vi "rs3_decode_streams.vi"(0 "Stream profile array":T2(array[cluster])=[{"ID"=42, "Profile"=521622968, "fps"=25, "RS Stream"=3, "RS Format"=10, "index"=2, "width"=1920, "height"=1080, "ppx"=0.0, "ppy"=0.0, "fx"=0.0, "fy"=0.0, "model"=0}, {"ID"=41, "Profile"=521634232, "fps"=25, "RS Stream"=3, "RS Format"=10, "index"=1, "width"=1920, "height"=1080, "ppx"=0.0, "ppy"=0.0, "fx"=0.0, "fy"=0.0, "model"=0}, {"ID"=42, "Profile"=521608632, "fps"=25, "RS Stream"=3, "RS Format"=9, "index"=2, "width"=1920, "height"=1080, "ppx"=951.85925, "ppy"=556.0496, "fx"=1428.9095, "fy"=1428.9095, "model"=4}, {"ID"=41, "Profile"=521617080, "fps"=25, "RS Stream"=3, "RS Format"=9, "index"=1, "width"=1920, "height"=1080, "ppx"=951.85925, "ppy"=556.0496, "fx"=1428.9095, "fy"=1428.9095, "model"=4}, {"ID"=41, "Profile"=521619128, "fps"=15, "RS Stream"=3, "RS Format"=10, "index"=1, "width"=1920, "height"=1080, "ppx"=0.0, "ppy"=0.0, "fx"=0.0, "fy"=0.0, "model"=0}, {"ID"=42, "Profile"=521623224, "fps"=15, "RS Stream"=3, "RS Format"=10, "index"=2, "width"=1920, "height"=1080, "ppx"=0.0, "ppy"=0.0, "fx"=0.0, "fy"=0.0, "model"=0}, {"ID"=42, "Profile"=521628088, "fps"=15, "RS Stream"=3, "RS Format"=9, "index"=2, "width"=1920, "height"=1080, "ppx"=951.85925, "ppy"=556.0496, "fx"=1428.9095, "fy"=1428.9095, "model"=4}, {"ID"=41, "Profile"=521627576, "fps"=15, "RS Stream"=3, "RS Format"=9, "index"=1, "width"=1920, "height"=1080, "ppx"=951.85925, "ppy"=556.0496, "fx"=1428.9095, "fy"=1428.9095, "model"=4}, {"ID"=41, "Profile"=521612728, "fps"=30, "RS Stream"=3, "RS Format"=14, "index"=0, "width"=1280, "height"=720, "ppx"=634.5728, "ppy"=370.69974, "fx"=952.6064, "fy"=952.6064, "model"=4}, {"ID"=41, "Profile"=521610424, "fps"=30, "RS Stream"=3, "RS Format"=10, "index"=0, "width"=1280, "height"=720, "ppx"=0.0, "ppy"=0.0, "fx"=0.0, "fy"=0.0, "model"=0}, {"ID"=42, "Profile"=521615544, "fps"=30, "RS Stream"=3, "RS Format"=9, "index"=2, "width"=1280, "height"=720, "ppx"=634.5728, "ppy"=370.69974, "fx"=952.6064, "fy"=952.6064, "model"=4}, {"ID"=41, "Profile"=521320344, "fps"=30, "RS Stream"=3, "RS Format"=9, "index"=1, "width"=1280, "height"=720, "ppx"=634.5728, "ppy"=370.69974, "fx"=952.6064, "fy"=952.6064, "model"=4}, {"ID"=41, "Profile"=521614520, "fps"=30, "RS Stream"=3, "RS Format"=8, "index"=0, "width"=1280, "height"=720, "ppx"=634.5728, "ppy"=370.69974, "fx"=952.6064, "fy"=952.6064, "model"=4}, {"ID"=41, "Profile"=521605816, "fps"=30, "RS Stream"=3, "RS Format"=7, "index"=0, "width"=1280, "height"=720, "ppx"=634.5728, "ppy"=370.69974, "fx"=952.6064, "fy"=952.6064, "model"=4}, {"ID"=41, "Profile"=521607608, "fps"=30, "RS Stream"=3, "RS Format"=6, "index"=0, "width"=1280, "height"=720, "ppx"=634.5728, "ppy"=370.69974, "fx"=952.6064, "fy"=952.6064, "model"=4}, {"ID"=41, "Profile"=521605560, "fps"=30, "RS Stream"=3, "RS Format"=5, "index"=0, "width"=1280, "height"=720, "ppx"=634.5728, "ppy"=370.69974, "fx"=952.6064, "fy"=952.6064, "model"=4}, {"ID"=41, "Profile"=521609912, "fps"=15, "RS Stream"=3, "RS Format"=14, "index"=0, "width"=1280, "height"=720, "ppx"=634.5728, "ppy"=370.69974, "fx"=952.6064, "fy"=952.6064, "model"=4}, {"ID"=41, "Profile"=521606584, "fps"=15, "RS Stream"=3, "RS Format"=10, "index"=0, "width"=1280, "height"=720, "ppx"=0.0, "ppy"=0.0, "fx"=0.0, "fy"=0.0, "model"=0}, {"ID"=41, "Profile"=521310872, "fps"=15, "RS Stream"=3, "RS Format"=9, "index"=1, "width"=1280, "height"=720, "ppx"=634.5728, "ppy"=370.69974, "fx"=952.6064, "fy"=952.6064, "model"=4}, {"ID"=42, "Profile"=521616824, "fps"=15, "RS Stream"=3, "RS Format"=9, "index"=2, "width"=1280, "height"=720, "ppx"=634.5728, "ppy"=370.69974, "fx"=952.6064, "fy"=952.6064, "model"=4}, {"ID"=41, "Profile"=521604024, "fps"=15, "RS Stream"=3, "RS Format"=8, "index"=0, "width"=1280, "height"=720, "ppx"=634.5728, "ppy"=370.69974, "fx"=952.6064, "fy"=952.6064, "model"=4}, {"ID"=41, "Profile"=521612984, "fps"=15, "RS Stream"=3, "RS Format"=7, "index"=0, "width"=1280, "height"=720, "ppx"=634.5728, "ppy"=370.69974, "fx"=952.6064, "fy"=952.6064, "model"=4}, {"ID"=41, "Profile"=521610168, "fps"=15, "RS Stream"=3, "RS Format"=6, "index"=0, "width"=1280, "height"=720, "ppx"=634.5728, "ppy"=370.69974, "fx"=952.6064, "fy"=952.6064, "model"=4}, {"ID"=41, "Profile"=521604536, "fps"=15, "RS Stream"=3, "RS Format"=5, "index"=0, "width"=1280, "height"=720, "ppx"=634.5728, "ppy"=370.69974, "fx"=952.6064, "fy"=952.6064, "model"=4}, {"ID"=41, "Profile"=521617848, "fps"=6, "RS Stream"=3, "RS Format"=14, "index"=0, "width"=1280, "height"=720, "ppx"=634.5728, "ppy"=370.69974, "fx"=952.6064, "fy"=952.6064, "model"=4}, {"ID"=41, "Profile"=521613752, "fps"=6, "RS Stream"=3, "RS Format"=10, "index"=0, "width"=1280, "height"=720, "ppx"=0.0, "ppy"=0.0, "fx"=0.0, "fy"=0.0, "model"=0}, {"ID"=41, "Profile"=521320600, "fps"=6, "RS Stream"=3, "RS Format"=9, "index"=1, "width"=1280, "height"=720, "ppx"=634.5728, "ppy"=370.69974, "fx"=952.6064, "fy"=952.6064, "model"=4}, {"ID"=42, "Profile"=521608888, "fps"=6, "RS Stream"=3, "RS Format"=9, "index"=2, "width"=1280, "height"=720, "ppx"=634.5728, "ppy"=370.69974, "fx"=952.6064, "fy"=952.6064, "model"=4}, {"ID"=41, "Profile"=521613240, "fps"=6, "RS Stream"=3, "RS Format"=8, "index"=0, "width"=1280, "height"=720, "ppx"=634.5728, "ppy"=370.69974, "fx"=952.6064, "fy"=952.6064, "model"=4}, {"ID"=41, "Profile"=521611704, "fps"=6, "RS Stream"=3, "RS Format"=7, "index"=0, "width"=1280, "height"=720, "ppx"=634.5728, "ppy"=370.69974, "fx"=952.6064, "fy"=952.6064, "model"=4}, {"ID"=41, "Profile"=521601720, "fps"=6, "RS Stream"=3, "RS Format"=6, "index"=0, "width"=1280, "height"=720, "ppx"=634.5728, "ppy"=370.69974, "fx"=952.6064, "fy"=952.6064, "model"=4}, {"ID"=41, "Profile"=521617336, "fps"=6, "RS Stream"=3, "RS Format"=5, "index"=0, "width"=1280, "height"=720, "ppx"=634.5728, "ppy"=370.69974, "fx"=952.6064, "fy"=952.6064, "model"=4}, {"ID"=41, "Profile"=521622712, "fps"=25, "RS Stream"=3, "RS Format"=10, "index"=1, "width"=960, "height"=540, "ppx"=0.0, "ppy"=0.0, "fx"=0.0, "fy"=0.0, "model"=0}, {"ID"=42, "Profile"=521633976, "fps"=25, "RS Stream"=3, "RS Format"=10, "index"=2, "width"=960, "height"=540, "ppx"=0.0, "ppy"=0.0, "fx"=0.0, "fy"=0.0, "model"=0}, {"ID"=42, "Profile"=521624504, "fps"=15, "RS Stream"=3, "RS Format"=10, "index"=2, "width"=960, "height"=540, "ppx"=0.0, "ppy"=0.0, "fx"=0.0, "fy"=0.0, "model"=0}, {"ID"=41, "Profile"=521622456, "fps"=15, "RS Stream"=3, "RS Format"=10, "index"=1, "width"=960, "height"=540, "ppx"=0.0, "ppy"=0.0, "fx"=0.0, "fy"=0.0, "model"=0}, {"ID"=41, "Profile"=521352856, "fps"=90, "RS Stream"=3, "RS Format"=14, "index"=0, "width"=848, "height"=480, "ppx"=420.38187, "ppy"=247.13316, "fx"=635.0709, "fy"=635.0709, "model"=4}, {"ID"=41, "Profile"=521351320, "fps"=90, "RS Stream"=3, "RS Format"=10, "index"=0, "width"=848, "height"=480, "ppx"=0.0, "ppy"=0.0, "fx"=0.0, "fy"=0.0, "model"=0}, {"ID"=41, "Profile"=521306776, "fps"=90, "RS Stream"=3, "RS Format"=9, "index"=1, "width"=848, "height"=480, "ppx"=420.38187, "ppy"=247.13316, "fx"=635.0709, "fy"=635.0709, "model"=4}, {"ID"=42, "Profile"=521614776, "fps"=90, "RS Stream"=3, "RS Format"=9, "index"=2, "width"=848, "height"=480, "ppx"=420.38187, "ppy"=247.13316, "fx"=635.0709, "fy"=635.0709, "model"=4}, {"ID"=41, "Profile"=521353624, "fps"=90, "RS Stream"=3, "RS Format"=8, "index"=0, "width"=848, "height"=480, "ppx"=420.38187, "ppy"=247.13316, "fx"=635.0709, "fy"=635.0709, "model"=4}, {"ID"=41, "Profile"=521339544, "fps"=90, "RS Stream"=3, "RS Format"=7, "index"=0, "width"=848, "height"=480, "ppx"=420.38187, "ppy"=247.13316, "fx"=635.0709, "fy"=635.0709, "model"=4}, {"ID"=41, "Profile"=521353368, "fps"=90, "RS Stream"=3, "RS Format"=6, "index"=0, "width"=848, "height"=480, "ppx"=420.38187, "ppy"=247.13316, "fx"=635.0709, "fy"=635.0709, "model"=4}, {"ID"=41, "Profile"=521351064, "fps"=90, "RS Stream"=3, "RS Format"=5, "index"=0, "width"=848, "height"=480, "ppx"=420.38187, "ppy"=247.13316, "fx"=635.0709, "fy"=635.0709, "model"=4}, {"ID"=41, "Profile"=521342104, "fps"=60, "RS Stream"=3, "RS Format"=14, "index"=0, "width"=848, "height"=480, "ppx"=420.38187, "ppy"=247.13316, "fx"=635.0709, "fy"=635.0709, "model"=4}, {"ID"=41, "Profile"=521341848, "fps"=60, "RS Stream"=3, "RS Format"=10, "index"=0, "width"=848, "height"=480, "ppx"=0.0, "ppy"=0.0, "fx"=0.0, "fy"=0.0, "model"=0}, {"ID"=42, "Profile"=521611960, "fps"=60, "RS Stream"=3, "RS Format"=9, "index"=2, "width"=848, "height"=480, "ppx"=420.38187, "ppy"=247.13316, "fx"=635.0709, "fy"=635.0709, "model"=4}, {"ID"=41, "Profile"=521310360, "fps"=60, "RS Stream"=3, "RS Format"=9, "index"=1, "width"=848, "height"=480, "ppx"=420.38187, "ppy"=247.13316, "fx"=635.0709, "fy"=635.0709, "model"=4}, {"ID"=41, "Profile"=521343384, "fps"=60, "RS Stream"=3, "RS Format"=8, "index"=0, "width"=848, "height"=480, "ppx"=420.38187, "ppy"=247.13316, "fx"=635.0709, "fy"=635.0709, "model"=4}, {"ID"=41, "Profile"=521342360, "fps"=60, "RS Stream"=3, "RS Format"=7, "index"=0, "width"=848, "height"=480, "ppx"=420.38187, "ppy"=247.13316, "fx"=635.0709, "fy"=635.0709, "model"=4}, {"ID"=41, "Profile"=521342616, "fps"=60, "RS Stream"=3, "RS Format"=6, "index"=0, "width"=848, "height"=480, "ppx"=420.38187, "ppy"=247.13316, "fx"=635.0709, "fy"=635.0709, "model"=4}, {"ID"=41, "Profile"=521354136, "fps"=60, "RS Stream"=3, "RS Format"=5, "index"=0, "width"=848, "height"=480, "ppx"=420.38187, "ppy"=247.13316, "fx"=635.0709, "fy"=635.0709, "model"=4}, {"ID"=41, "Profile"=521616056, "fps"=30, "RS Stream"=3, "RS Format"=14, "index"=0, "width"=848, "height"=480, "ppx"=420.38187, "ppy"=247.13316, "fx"=635.0709, "fy"=635.0709, "model"=4}, {"ID"=41, "Profile"=514733800, "fps"=30, "RS Stream"=3, "RS Format"=10, "index"=0, "width"=848, "height"=480, "ppx"=0.0, "ppy"=0.0, "fx"=0.0, "fy"=0.0, "model"=0}, {"ID"=42, "Profile"=521609144, "fps"=30, "RS Stream"=3, "RS Format"=9, "index"=2, "width"=848, "height"=480, "ppx"=420.38187, "ppy"=247.13316, "fx"=635.0709, "fy"=635.0709, "model"=4}, {"ID"=41, "Profile"=521310616, "fps"=30, "RS Stream"=3, "RS Format"=9, "index"=1, "width"=848, "height"=480, "ppx"=420.38187, "ppy"=247.13316, "fx"=635.0709, "fy"=635.0709, "model"=4}, {"ID"=41, "Profile"=521606840, "fps"=30, "RS Stream"=3, "RS Format"=8, "index"=0, "width"=848, "height"=480, "ppx"=420.38187, "ppy"=247.13316, "fx"=635.0709, "fy"=635.0709, "model"=4}, {"ID"=41, "Profile"=521603256, "fps"=30, "RS Stream"=3, "RS Format"=7, "index"=0, "width"=848, "height"=480, "ppx"=420.38187, "ppy"=247.13316, "fx"=635.0709, "fy"=635.0709, "model"=4}, {"ID"=41, "Profile"=521612472, "fps"=30, "RS Stream"=3, "RS Format"=6, "index"=0, "width"=848, "height"=480, "ppx"=420.38187, "ppy"=247.13316, "fx"=635.0709, "fy"=635.0709, "model"=4}, {"ID"=41, "Profile"=521343640, "fps"=30, "RS Stream"=3, "RS Format"=5, "index"=0, "width"=848, "height"=480, "ppx"=420.38187, "ppy"=247.13316, "fx"=635.0709, "fy"=635.0709, "model"=4}, {"ID"=41, "Profile"=521609400, "fps"=15, "RS Stream"=3, "RS Format"=14, "index"=0, "width"=848, "height"=480, "ppx"=420.38187, "ppy"=247.13316, "fx"=635.0709, "fy"=635.0709, "model"=4}, {"ID"=41, "Profile"=521606328, "fps"=15, "RS Stream"=3, "RS Format"=10, "index"=0, "width"=848, "height"=480, "ppx"=0.0, "ppy"=0.0, "fx"=0.0, "fy"=0.0, "model"=0}, {"ID"=41, "Profile"=521317272, "fps"=15, "RS Stream"=3, "RS Format"=9, "index"=1, "width"=848, "height"=480, "ppx"=420.38187, "ppy"=247.13316, "fx"=635.0709, "fy"=635.0709, "model"=4}, {"ID"=42, "Profile"=521615288, "fps"=15, "RS Stream"=3, "RS Format"=9, "index"=2, "width"=848, "height"=480, "ppx"=420.38187, "ppy"=247.13316, "fx"=635.0709, "fy"=635.0709, "model"=4}, {"ID"=41, "Profile"=521603512, "fps"=15, "RS Stream"=3, "RS Format"=8, "index"=0, "width"=848, "height"=480, "ppx"=420.38187, "ppy"=247.13316, "fx"=635.0709, "fy"=635.0709, "model"=4}, {"ID"=41, "Profile"=521602744, "fps"=15, "RS Stream"=3, "RS Format"=7, "index"=0, "width"=848, "height"=480, "ppx"=420.38187, "ppy"=247.13316, "fx"=635.0709, "fy"=635.0709, "model"=4}, {"ID"=41, "Profile"=521607096, "fps"=15, "RS Stream"=3, "RS Format"=6, "index"=0, "width"=848, "height"=480, "ppx"=420.38187, "ppy"=247.13316, "fx"=635.0709, "fy"=635.0709, "model"=4}, {"ID"=41, "Profile"=521617592, "fps"=15, "RS Stream"=3, "RS Format"=5, "index"=0, "width"=848, "height"=480, "ppx"=420.38187, "ppy"=247.13316, "fx"=635.0709, "fy"=635.0709, "model"=4}, {"ID"=41, "Profile"=521603768, "fps"=6, "RS Stream"=3, "RS Format"=14, "index"=0, "width"=848, "height"=480, "ppx"=420.38187, "ppy"=247.13316, "fx"=635.0709, "fy"=635.0709, "model"=4}, {"ID"=41, "Profile"=521604280, "fps"=6, "RS Stream"=3, "RS Format"=10, "index"=0, "width"=848, "height"=480, "ppx"=0.0, "ppy"=0.0, "fx"=0.0, "fy"=0.0, "model"=0}, {"ID"=42, "Profile"=521616568, "fps"=6, "RS Stream"=3, "RS Format"=9, "index"=2, "width"=848, "height"=480, "ppx"=420.38187, "ppy"=247.13316, "fx"=635.0709, "fy"=635.0709, "model"=4}, {"ID"=41, "Profile"=521315992, "fps"=6, "RS Stream"=3, "RS Format"=9, "index"=1, "width"=848, "height"=480, "ppx"=420.38187, "ppy"=247.13316, "fx"=635.0709, "fy"=635.0709, "model"=4}, {"ID"=41, "Profile"=521607864, "fps"=6, "RS Stream"=3, "RS Format"=8, "index"=0, "width"=848, "height"=480, "ppx"=420.38187, "ppy"=247.13316, "fx"=635.0709, "fy"=635.0709, "model"=4}, {"ID"=41, "Profile"=521616312, "fps"=6, "RS Stream"=3, "RS Format"=7, "index"=0, "width"=848, "height"=480, "ppx"=420.38187, "ppy"=247.13316, "fx"=635.0709, "fy"=635.0709, "model"=4}, {"ID"=41, "Profile"=521615800, "fps"=6, "RS Stream"=3, "RS Format"=6, "index"=0, "width"=848, "height"=480, "ppx"=420.38187, "ppy"=247.13316, "fx"=635.0709, "fy"=635.0709, "model"=4}, {"ID"=41, "Profile"=521610680, "fps"=6, "RS Stream"=3, "RS Format"=5, "index"=0, "width"=848, "height"=480, "ppx"=420.38187, "ppy"=247.13316, "fx"=635.0709, "fy"=635.0709, "model"=4}, {"ID"=41, "Profile"=521348504, "fps"=90, "RS Stream"=3, "RS Format"=14, "index"=0, "width"=640, "height"=480, "ppx"=316.38187, "ppy"=247.13316, "fx"=635.0709, "fy"=635.0709, "model"=4}, {"ID"=41, "Profile"=521354904, "fps"=90, "RS Stream"=3, "RS Format"=10, "index"=0, "width"=640, "height"=480, "ppx"=0.0, "ppy"=0.0, "fx"=0.0, "fy"=0.0, "model"=0}, {"ID"=42, "Profile"=521605304, "fps"=90, "RS Stream"=3, "RS Format"=9, "index"=2, "width"=640, "height"=480, "ppx"=316.38187, "ppy"=247.13316, "fx"=635.0709, "fy"=635.0709, "model"=4}, {"ID"=41, "Profile"=521322648, "fps"=90, "RS Stream"=3, "RS Format"=9, "index"=1, "width"=640, "height"=480, "ppx"=316.38187, "ppy"=247.13316, "fx"=635.0709, "fy"=635.0709, "model"=4}, {"ID"=41, "Profile"=521340056, "fps"=90, "RS Stream"=3, "RS Format"=8, "index"=0, "width"=640, "height"=480, "ppx"=316.38187, "ppy"=247.13316, "fx"=635.0709, "fy"=635.0709, "model"=4}, {"ID"=41, "Profile"=521355672, "fps"=90, "RS Stream"=3, "RS Format"=7, "index"=0, "width"=640, "height"=480, "ppx"=316.38187, "ppy"=247.13316, "fx"=635.0709, "fy"=635.0709, "model"=4}, {"ID"=41, "Profile"=521352088, "fps"=90, "RS Stream"=3, "RS Format"=6, "index"=0, "width"=640, "height"=480, "ppx"=316.38187, "ppy"=247.13316, "fx"=635.0709, "fy"=635.0709, "model"=4}, {"ID"=41, "Profile"=521351576, "fps"=90, "RS Stream"=3, "RS Format"=5, "index"=0, "width"=640, "height"=480, "ppx"=316.38187, "ppy"=247.13316, "fx"=635.0709, "fy"=635.0709, "model"=4}, {"ID"=41, "Profile"=521352344, "fps"=60, "RS Stream"=3, "RS Format"=14, "index"=0, "width"=640, "height"=480, "ppx"=316.38187, "ppy"=247.13316, "fx"=635.0709, "fy"=635.0709, "model"=4}, {"ID"=41, "Profile"=521354648, "fps"=60, "RS Stream"=3, "RS Format"=10, "index"=0, "width"=640, "height"=480, "ppx"=0.0, "ppy"=0.0, "fx"=0.0, "fy"=0.0, "model"=0}, {"ID"=41, "Profile"=521320088, "fps"=60, "RS Stream"=3, "RS Format"=9, "index"=1, "width"=640, "height"=480, "ppx"=316.38187, "ppy"=247.13316, "fx"=635.0709, "fy"=635.0709, "model"=4}, {"ID"=42, "Profile"=521615032, "fps"=60, "RS Stream"=3, "RS Format"=9, "index"=2, "width"=640, "height"=480, "ppx"=316.38187, "ppy"=247.13316, "fx"=635.0709, "fy"=635.0709, "model"=4}, {"ID"=41, "Profile"=521340312, "fps"=60, "RS Stream"=3, "RS Format"=8, "index"=0, "width"=640, "height"=480, "ppx"=316.38187, "ppy"=247.13316, "fx"=635.0709, "fy"=635.0709, "model"=4}, {"ID"=41, "Profile"=521342872, "fps"=60, "RS Stream"=3, "RS Format"=7, "index"=0, "width"=640, "height"=480, "ppx"=316.38187, "ppy"=247.13316, "fx"=635.0709, "fy"=635.0709, "model"=4}, {"ID"=41, "Profile"=521346200, "fps"=60, "RS Stream"=3, "RS Format"=6, "index"=0, "width"=640, "height"=480, "ppx"=316.38187, "ppy"=247.13316, "fx"=635.0709, "fy"=635.0709, "model"=4}, {"ID"=41, "Profile"=521345944, "fps"=60, "RS Stream"=3, "RS Format"=5, "index"=0, "width"=640, "height"=480, "ppx"=316.38187, "ppy"=247.13316, "fx"=635.0709, "fy"=635.0709, "model"=4}, {"ID"=41, "Profile"=521344408, "fps"=30, "RS Stream"=3, "RS Format"=14, "index"=0, "width"=640, "height"=480, "ppx"=316.38187, "ppy"=247.13316, "fx"=635.0709, "fy"=635.0709, "model"=4}, {"ID"=41, "Profile"=521348248, "fps"=30, "RS Stream"=3, "RS Format"=10, "index"=0, "width"=640, "height"=480, "ppx"=0.0, "ppy"=0.0, "fx"=0.0, "fy"=0.0, "model"=0}, {"ID"=41, "Profile"=521309592, "fps"=30, "RS Stream"=3, "RS Format"=9, "index"=1, "width"=640, "height"=480, "ppx"=316.38187, "ppy"=247.13316, "fx"=635.0709, "fy"=635.0709, "model"=4}, {"ID"=42, "Profile"=521607352, "fps"=30, "RS Stream"=3, "RS Format"=9, "index"=2, "width"=640, "height"=480, "ppx"=316.38187, "ppy"=247.13316, "fx"=635.0709, "fy"=635.0709, "model"=4}, {"ID"=41, "Profile"=521352600, "fps"=30, "RS Stream"=3, "RS Format"=8, "index"=0, "width"=640, "height"=480, "ppx"=316.38187, "ppy"=247.13316, "fx"=635.0709, "fy"=635.0709, "model"=4}, {"ID"=41, "Profile"=521344664, "fps"=30, "RS Stream"=3, "RS Format"=7, "index"=0, "width"=640, "height"=480, "ppx"=316.38187, "ppy"=247.13316, "fx"=635.0709, "fy"=635.0709, "model"=4}, {"ID"=41, "Profile"=521344920, "fps"=30, "RS Stream"=3, "RS Format"=6, "index"=0, "width"=640, "height"=480, "ppx"=316.38187, "ppy"=247.13316, "fx"=635.0709, "fy"=635.0709, "model"=4}, {"ID"=41, "Profile"=521350296, "fps"=30, "RS Stream"=3, "RS Format"=5, "index"=0, "width"=640, "height"=480, "ppx"=316.38187, "ppy"=247.13316, "fx"=635.0709, "fy"=635.0709, "model"=4}, {"ID"=41, "Profile"=521355160, "fps"=15, "RS Stream"=3, "RS Format"=14, "index"=0, "width"=640, "height"=480, "ppx"=316.38187, "ppy"=247.13316, "fx"=635.0709, "fy"=635.0709, "model"=4}, {"ID"=41, "Profile"=521341592, "fps"=15, "RS Stream"=3, "RS Format"=10, "index"=0, "width"=640, "height"=480, "ppx"=0.0, "ppy"=0.0, "fx"=0.0, "fy"=0.0, "model"=0}, {"ID"=41, "Profile"=521321368, "fps"=15, "RS Stream"=3, "RS Format"=9, "index"=1, "width"=640, "height"=480, "ppx"=316.38187, "ppy"=247.13316, "fx"=635.0709, "fy"=635.0709, "model"=4}, {"ID"=42, "Profile"=521608120, "fps"=15, "RS Stream"=3, "RS Format"=9, "index"=2, "width"=640, "height"=480, "ppx"=316.38187, "ppy"=247.13316, "fx"=635.0709, "fy"=635.0709, "model"=4}, {"ID"=41, "Profile"=521346968, "fps"=15, "RS Stream"=3, "RS Format"=8, "index"=0, "width"=640, "height"=480, "ppx"=316.38187, "ppy"=247.13316, "fx"=635.0709, "fy"=635.0709, "model"=4}, {"ID"=41, "Profile"=521348760, "fps"=15, "RS Stream"=3, "RS Format"=7, "index"=0, "width"=640, "height"=480, "ppx"=316.38187, "ppy"=247.13316, "fx"=635.0709, "fy"=635.0709, "model"=4}, {"ID"=41, "Profile"=521339800, "fps"=15, "RS Stream"=3, "RS Format"=6, "index"=0, "width"=640, "height"=480, "ppx"=316.38187, "ppy"=247.13316, "fx"=635.0709, "fy"=635.0709, "model"=4}, {"ID"=41, "Profile"=521350808, "fps"=15, "RS Stream"=3, "RS Format"=5, "index"=0, "width"=640, "height"=480, "ppx"=316.38187, "ppy"=247.13316, "fx"=635.0709, "fy"=635.0709, "model"=4}, {"ID"=41, "Profile"=521349016, "fps"=6, "RS Stream"=3, "RS Format"=14, "index"=0, "width"=640, "height"=480, "ppx"=316.38187, "ppy"=247.13316, "fx"=635.0709, "fy"=635.0709, "model"=4}, {"ID"=41, "Profile"=521346456, "fps"=6, "RS Stream"=3, "RS Format"=10, "index"=0, "width"=640, "height"=480, "ppx"=0.0, "ppy"=0.0, "fx"=0.0, "fy"=0.0, "model"=0}, {"ID"=42, "Profile"=521608376, "fps"=6, "RS Stream"=3, "RS Format"=9, "index"=2, "width"=640, "height"=480, "ppx"=316.38187, "ppy"=247.13316, "fx"=635.0709, "fy"=635.0709, "model"=4}, {"ID"=41, "Profile"=521313176, "fps"=6, "RS Stream"=3, "RS Format"=9, "index"=1, "width"=640, "height"=480, "ppx"=316.38187, "ppy"=247.13316, "fx"=635.0709, "fy"=635.0709, "model"=4}, {"ID"=41, "Profile"=521343128, "fps"=6, "RS Stream"=3, "RS Format"=8, "index"=0, "width"=640, "height"=480, "ppx"=316.38187, "ppy"=247.13316, "fx"=635.0709, "fy"=635.0709, "model"=4}, {"ID"=41, "Profile"=521349528, "fps"=6, "RS Stream"=3, "RS Format"=7, "index"=0, "width"=640, "height"=480, "ppx"=316.38187, "ppy"=247.13316, "fx"=635.0709, "fy"=635.0709, "model"=4}, {"ID"=41, "Profile"=521355416, "fps"=6, "RS Stream"=3, "RS Format"=6, "index"=0, "width"=640, "height"=480, "ppx"=316.38187, "ppy"=247.13316, "fx"=635.0709, "fy"=635.0709, "model"=4}, {"ID"=41, "Profile"=521349272, "fps"=6, "RS Stream"=3, "RS Format"=5, "index"=0, "width"=640, "height"=480, "ppx"=316.38187, "ppy"=247.13316, "fx"=635.0709, "fy"=635.0709, "model"=4}, {"ID"=41, "Profile"=521330840, "fps"=90, "RS Stream"=3, "RS Format"=14, "index"=0, "width"=640, "height"=360, "ppx"=317.2864, "ppy"=185.34987, "fx"=476.3032, "fy"=476.3032, "model"=4}, {"ID"=41, "Profile"=521330584, "fps"=90, "RS Stream"=3, "RS Format"=10, "index"=0, "width"=640, "height"=360, "ppx"=0.0, "ppy"=0.0, "fx"=0.0, "fy"=0.0, "model"=0}, {"ID"=41, "Profile"=521318296, "fps"=90, "RS Stream"=3, "RS Format"=9, "index"=1, "width"=640, "height"=360, "ppx"=317.2864, "ppy"=185.34987, "fx"=476.3032, "fy"=476.3032, "model"=4}, {"ID"=42, "Profile"=521609656, "fps"=90, "RS Stream"=3, "RS Format"=9, "index"=2, "width"=640, "height"=360, "ppx"=317.2864, "ppy"=185.34987, "fx"=476.3032, "fy"=476.3032, "model"=4}, {"ID"=41, "Profile"=521332120, "fps"=90, "RS Stream"=3, "RS Format"=8, "index"=0, "width"=640, "height"=360, "ppx"=317.2864, "ppy"=185.34987, "fx"=476.3032, "fy"=476.3032, "model"=4}, {"ID"=41, "Profile"=521331608, "fps"=90, "RS Stream"=3, "RS Format"=7, "index"=0, "width"=640, "height"=360, "ppx"=317.2864, "ppy"=185.34987, "fx"=476.3032, "fy"=476.3032, "model"=4}, {"ID"=41, "Profile"=521331864, "fps"=90, "RS Stream"=3, "RS Format"=6, "index"=0, "width"=640, "height"=360, "ppx"=317.2864, "ppy"=185.34987, "fx"=476.3032, "fy"=476.3032, "model"=4}, {"ID"=41, "Profile"=521326744, "fps"=90, "RS Stream"=3, "RS Format"=5, "index"=0, "width"=640, "height"=360, "ppx"=317.2864, "ppy"=185.34987, "fx"=476.3032, "fy"=476.3032, "model"=4}, {"ID"=41, "Profile"=521333912, "fps"=60, "RS Stream"=3, "RS Format"=14, "index"=0, "width"=640, "height"=360, "ppx"=317.2864, "ppy"=185.34987, "fx"=476.3032, "fy"=476.3032, "model"=4}, {"ID"=41, "Profile"=521333144, "fps"=60, "RS Stream"=3, "RS Format"=10, "index"=0, "width"=640, "height"=360, "ppx"=0.0, "ppy"=0.0, "fx"=0.0, "fy"=0.0, "model"=0}, {"ID"=42, "Profile"=521606072, "fps"=60, "RS Stream"=3, "RS Format"=9, "index"=2, "width"=640, "height"=360, "ppx"=317.2864, "ppy"=185.34987, "fx"=476.3032, "fy"=476.3032, "model"=4}, {"ID"=41, "Profile"=521321112, "fps"=60, "RS Stream"=3, "RS Format"=9, "index"=1, "width"=640, "height"=360, "ppx"=317.2864, "ppy"=185.34987, "fx"=476.3032, "fy"=476.3032, "model"=4}, {"ID"=41, "Profile"=521340824, "fps"=60, "RS Stream"=3, "RS Format"=8, "index"=0, "width"=640, "height"=360, "ppx"=317.2864, "ppy"=185.34987, "fx"=476.3032, "fy"=476.3032, "model"=4}, {"ID"=41, "Profile"=521353880, "fps"=60, "RS Stream"=3, "RS Format"=7, "index"=0, "width"=640, "height"=360, "ppx"=317.2864, "ppy"=185.34987, "fx"=476.3032, "fy"=476.3032, "model"=4}, {"ID"=41, "Profile"=521350552, "fps"=60, "RS Stream"=3, "RS Format"=6, "index"=0, "width"=640, "height"=360, "ppx"=317.2864, "ppy"=185.34987, "fx"=476.3032, "fy"=476.3032, "model"=4}, {"ID"=41, "Profile"=521332888, "fps"=60, "RS Stream"=3, "RS Format"=5, "index"=0, "width"=640, "height"=360, "ppx"=317.2864, "ppy"=185.34987, "fx"=476.3032, "fy"=476.3032, "model"=4}, {"ID"=41, "Profile"=521347224, "fps"=30, "RS Stream"=3, "RS Format"=14, "index"=0, "width"=640, "height"=360, "ppx"=317.2864, "ppy"=185.34987, "fx"=476.3032, "fy"=476.3032, "model"=4}, {"ID"=41, "Profile"=521349784, "fps"=30, "RS Stream"=3, "RS Format"=10, "index"=0, "width"=640, "height"=360, "ppx"=0.0, "ppy"=0.0, "fx"=0.0, "fy"=0.0, "model"=0}, {"ID"=42, "Profile"=521604792, "fps"=30, "RS Stream"=3, "RS Format"=9, "index"=2, "width"=640, "height"=360, "ppx"=317.2864, "ppy"=185.34987, "fx"=476.3032, "fy"=476.3032, "model"=4}, {"ID"=41, "Profile"=521319064, "fps"=30, "RS Stream"=3, "RS Format"=9, "index"=1, "width"=640, "height"=360, "ppx"=317.2864, "ppy"=185.34987, "fx"=476.3032, "fy"=476.3032, "model"=4}, {"ID"=41, "Profile"=521351832, "fps"=30, "RS Stream"=3, "RS Format"=8, "index"=0, "width"=640, "height"=360, "ppx"=317.2864, "ppy"=185.34987, "fx"=476.3032, "fy"=476.3032, "model"=4}, {"ID"=41, "Profile"=521347480, "fps"=30, "RS Stream"=3, "RS Format"=7, "index"=0, "width"=640, "height"=360, "ppx"=317.2864, "ppy"=185.34987, "fx"=476.3032, "fy"=476.3032, "model"=4}, {"ID"=41, "Profile"=521350040, "fps"=30, "RS Stream"=3, "RS Format"=6, "index"=0, "width"=640, "height"=360, "ppx"=317.2864, "ppy"=185.34987, "fx"=476.3032, "fy"=476.3032, "model"=4}, {"ID"=41, "Profile"=521345432, "fps"=30, "RS Stream"=3, "RS Format"=5, "index"=0, "width"=640, "height"=360, "ppx"=317.2864, "ppy"=185.34987, "fx"=476.3032, "fy"=476.3032, "model"=4}, {"ID"=41, "Profile"=521343896, "fps"=15, "RS Stream"=3, "RS Format"=14, "index"=0, "width"=640, "height"=360, "ppx"=317.2864, "ppy"=185.34987, "fx"=476.3032, "fy"=476.3032, "model"=4}, {"ID"=41, "Profile"=521340568, "fps"=15, "RS Stream"=3, "RS Format"=10, "index"=0, "width"=640, "height"=360, "ppx"=0.0, "ppy"=0.0, "fx"=0.0, "fy"=0.0, "model"=0}, {"ID"=41, "Profile"=521319320, "fps"=15, "RS Stream"=3, "RS Format"=9, "index"=1, "width"=640, "height"=360, "ppx"=317.2864, "ppy"=185.34987, "fx"=476.3032, "fy"=476.3032, "model"=4}, {"ID"=42, "Profile"=521613496, "fps"=15, "RS Stream"=3, "RS Format"=9, "index"=2, "width"=640, "height"=360, "ppx"=317.2864, "ppy"=185.34987, "fx"=476.3032, "fy"=476.3032, "model"=4}, {"ID"=41, "Profile"=521347736, "fps"=15, "RS Stream"=3, "RS Format"=8, "index"=0, "width"=640, "height"=360, "ppx"=317.2864, "ppy"=185.34987, "fx"=476.3032, "fy"=476.3032, "model"=4}, {"ID"=41, "Profile"=521345176, "fps"=15, "RS Stream"=3, "RS Format"=7, "index"=0, "width"=640, "height"=360, "ppx"=317.2864, "ppy"=185.34987, "fx"=476.3032, "fy"=476.3032, "model"=4}, {"ID"=41, "Profile"=521345688, "fps"=15, "RS Stream"=3, "RS Format"=6, "index"=0, "width"=640, "height"=360, "ppx"=317.2864, "ppy"=185.34987, "fx"=476.3032, "fy"=476.3032, "model"=4}, {"ID"=41, "Profile"=521347992, "fps"=15, "RS Stream"=3, "RS Format"=5, "index"=0, "width"=640, "height"=360, "ppx"=317.2864, "ppy"=185.34987, "fx"=476.3032, "fy"=476.3032, "model"=4}, {"ID"=41, "Profile"=521354392, "fps"=6, "RS Stream"=3, "RS Format"=14, "index"=0, "width"=640, "height"=360, "ppx"=317.2864, "ppy"=185.34987, "fx"=476.3032, "fy"=476.3032, "model"=4}, {"ID"=41, "Profile"=521341080, "fps"=6, "RS Stream"=3, "RS Format"=10, "index"=0, "width"=640, "height"=360, "ppx"=0.0, "ppy"=0.0, "fx"=0.0, "fy"=0.0, "model"=0}, {"ID"=42, "Profile"=521611448, "fps"=6, "RS Stream"=3, "RS Format"=9, "index"=2, "width"=640, "height"=360, "ppx"=317.2864, "ppy"=185.34987, "fx"=476.3032, "fy"=476.3032, "model"=4}, {"ID"=41, "Profile"=521314200, "fps"=6, "RS Stream"=3, "RS Format"=9, "index"=1, "width"=640, "height"=360, "ppx"=317.2864, "ppy"=185.34987, "fx"=476.3032, "fy"=476.3032, "model"=4}, {"ID"=41, "Profile"=521341336, "fps"=6, "RS Stream"=3, "RS Format"=8, "index"=0, "width"=640, "height"=360, "ppx"=317.2864, "ppy"=185.34987, "fx"=476.3032, "fy"=476.3032, "model"=4}, {"ID"=41, "Profile"=521344152, "fps"=6, "RS Stream"=3, "RS Format"=7, "index"=0, "width"=640, "height"=360, "ppx"=317.2864, "ppy"=185.34987, "fx"=476.3032, "fy"=476.3032, "model"=4}, {"ID"=41, "Profile"=521346712, "fps"=6, "RS Stream"=3, "RS Format"=6, "index"=0, "width"=640, "height"=360, "ppx"=317.2864, "ppy"=185.34987, "fx"=476.3032, "fy"=476.3032, "model"=4}, {"ID"=41, "Profile"=521353112, "fps"=6, "RS Stream"=3, "RS Format"=5, "index"=0, "width"=640, "height"=360, "ppx"=317.2864, "ppy"=185.34987, "fx"=476.3032, "fy"=476.3032, "model"=4}, {"ID"=41, "Profile"=521325720, "fps"=90, "RS Stream"=3, "RS Format"=14, "index"=0, "width"=480, "height"=270, "ppx"=237.96481, "ppy"=139.0124, "fx"=357.2274, "fy"=357.2274, "model"=4}, {"ID"=41, "Profile"=521331096, "fps"=90, "RS Stream"=3, "RS Format"=10, "index"=0, "width"=480, "height"=270, "ppx"=0.0, "ppy"=0.0, "fx"=0.0, "fy"=0.0, "model"=0}, {"ID"=42, "Profile"=521612216, "fps"=90, "RS Stream"=3, "RS Format"=9, "index"=2, "width"=480, "height"=270, "ppx"=237.96481, "ppy"=139.0124, "fx"=357.2274, "fy"=357.2274, "model"=4}, {"ID"=41, "Profile"=521312152, "fps"=90, "RS Stream"=3, "RS Format"=9, "index"=1, "width"=480, "height"=270, "ppx"=237.96481, "ppy"=139.0124, "fx"=357.2274, "fy"=357.2274, "model"=4}, {"ID"=41, "Profile"=521327768, "fps"=90, "RS Stream"=3, "RS Format"=8, "index"=0, "width"=480, "height"=270, "ppx"=237.96481, "ppy"=139.0124, "fx"=357.2274, "fy"=357.2274, "model"=4}, {"ID"=41, "Profile"=521336472, "fps"=90, "RS Stream"=3, "RS Format"=7, "index"=0, "width"=480, "height"=270, "ppx"=237.96481, "ppy"=139.0124, "fx"=357.2274, "fy"=357.2274, "model"=4}, {"ID"=41, "Profile"=521336728, "fps"=90, "RS Stream"=3, "RS Format"=6, "index"=0, "width"=480, "height"=270, "ppx"=237.96481, "ppy"=139.0124, "fx"=357.2274, "fy"=357.2274, "model"=4}, {"ID"=41, "Profile"=521326232, "fps"=90, "RS Stream"=3, "RS Format"=5, "index"=0, "width"=480, "height"=270, "ppx"=237.96481, "ppy"=139.0124, "fx"=357.2274, "fy"=357.2274, "model"=4}, {"ID"=41, "Profile"=521336984, "fps"=60, "RS Stream"=3, "RS Format"=14, "index"=0, "width"=480, "height"=270, "ppx"=237.96481, "ppy"=139.0124, "fx"=357.2274, "fy"=357.2274, "model"=4}, {"ID"=41, "Profile"=521328024, "fps"=60, "RS Stream"=3, "RS Format"=10, "index"=0, "width"=480, "height"=270, "ppx"=0.0, "ppy"=0.0, "fx"=0.0, "fy"=0.0, "model"=0}, {"ID"=41, "Profile"=521322904, "fps"=60, "RS Stream"=3, "RS Format"=9, "index"=1, "width"=480, "height"=270, "ppx"=237.96481, "ppy"=139.0124, "fx"=357.2274, "fy"=357.2274, "model"=4}, {"ID"=42, "Profile"=521603000, "fps"=60, "RS Stream"=3, "RS Format"=9, "index"=2, "width"=480, "height"=270, "ppx"=237.96481, "ppy"=139.0124, "fx"=357.2274, "fy"=357.2274, "model"=4}, {"ID"=41, "Profile"=521338264, "fps"=60, "RS Stream"=3, "RS Format"=8, "index"=0, "width"=480, "height"=270, "ppx"=237.96481, "ppy"=139.0124, "fx"=357.2274, "fy"=357.2274, "model"=4}, {"ID"=41, "Profile"=521337752, "fps"=60, "RS Stream"=3, "RS Format"=7, "index"=0, "width"=480, "height"=270, "ppx"=237.96481, "ppy"=139.0124, "fx"=357.2274, "fy"=357.2274, "model"=4}, {"ID"=41, "Profile"=521323416, "fps"=60, "RS Stream"=3, "RS Format"=6, "index"=0, "width"=480, "height"=270, "ppx"=237.96481, "ppy"=139.0124, "fx"=357.2274, "fy"=357.2274, "model"=4}, {"ID"=41, "Profile"=521337496, "fps"=60, "RS Stream"=3, "RS Format"=5, "index"=0, "width"=480, "height"=270, "ppx"=237.96481, "ppy"=139.0124, "fx"=357.2274, "fy"=357.2274, "model"=4}, {"ID"=41, "Profile"=521329816, "fps"=30, "RS Stream"=3, "RS Format"=14, "index"=0, "width"=480, "height"=270, "ppx"=237.96481, "ppy"=139.0124, "fx"=357.2274, "fy"=357.2274, "model"=4}, {"ID"=41, "Profile"=521328280, "fps"=30, "RS Stream"=3, "RS Format"=10, "index"=0, "width"=480, "height"=270, "ppx"=0.0, "ppy"=0.0, "fx"=0.0, "fy"=0.0, "model"=0}, {"ID"=42, "Profile"=521605048, "fps"=30, "RS Stream"=3, "RS Format"=9, "index"=2, "width"=480, "height"=270, "ppx"=237.96481, "ppy"=139.0124, "fx"=357.2274, "fy"=357.2274, "model"=4}, {"ID"=41, "Profile"=521316504, "fps"=30, "RS Stream"=3, "RS Format"=9, "index"=1, "width"=480, "height"=270, "ppx"=237.96481, "ppy"=139.0124, "fx"=357.2274, "fy"=357.2274, "model"=4}, {"ID"=41, "Profile"=521325464, "fps"=30, "RS Stream"=3, "RS Format"=8, "index"=0, "width"=480, "height"=270, "ppx"=237.96481, "ppy"=139.0124, "fx"=357.2274, "fy"=357.2274, "model"=4}, {"ID"=41, "Profile"=521325976, "fps"=30, "RS Stream"=3, "RS Format"=7, "index"=0, "width"=480, "height"=270, "ppx"=237.96481, "ppy"=139.0124, "fx"=357.2274, "fy"=357.2274, "model"=4}, {"ID"=41, "Profile"=521338520, "fps"=30, "RS Stream"=3, "RS Format"=6, "index"=0, "width"=480, "height"=270, "ppx"=237.96481, "ppy"=139.0124, "fx"=357.2274, "fy"=357.2274, "model"=4}, {"ID"=41, "Profile"=521332632, "fps"=30, "RS Stream"=3, "RS Format"=5, "index"=0, "width"=480, "height"=270, "ppx"=237.96481, "ppy"=139.0124, "fx"=357.2274, "fy"=357.2274, "model"=4}, {"ID"=41, "Profile"=521330328, "fps"=15, "RS Stream"=3, "RS Format"=14, "index"=0, "width"=480, "height"=270, "ppx"=237.96481, "ppy"=139.0124, "fx"=357.2274, "fy"=357.2274, "model"=4}, {"ID"=41, "Profile"=521328536, "fps"=15, "RS Stream"=3, "RS Format"=10, "index"=0, "width"=480, "height"=270, "ppx"=0.0, "ppy"=0.0, "fx"=0.0, "fy"=0.0, "model"=0}, {"ID"=41, "Profile"=521318808, "fps"=15, "RS Stream"=3, "RS Format"=9, "index"=1, "width"=480, "height"=270, "ppx"=237.96481, "ppy"=139.0124, "fx"=357.2274, "fy"=357.2274, "model"=4}, {"ID"=42, "Profile"=521610936, "fps"=15, "RS Stream"=3, "RS Format"=9, "index"=2, "width"=480, "height"=270, "ppx"=237.96481, "ppy"=139.0124, "fx"=357.2274, "fy"=357.2274, "model"=4}, {"ID"=41, "Profile"=521324440, "fps"=15, "RS Stream"=3, "RS Format"=8, "index"=0, "width"=480, "height"=270, "ppx"=237.96481, "ppy"=139.0124, "fx"=357.2274, "fy"=357.2274, "model"=4}, {"ID"=41, "Profile"=521328792, "fps"=15, "RS Stream"=3, "RS Format"=7, "index"=0, "width"=480, "height"=270, "ppx"=237.96481, "ppy"=139.0124, "fx"=357.2274, "fy"=357.2274, "model"=4}, {"ID"=41, "Profile"=521324184, "fps"=15, "RS Stream"=3, "RS Format"=6, "index"=0, "width"=480, "height"=270, "ppx"=237.96481, "ppy"=139.0124, "fx"=357.2274, "fy"=357.2274, "model"=4}, {"ID"=41, "Profile"=521323672, "fps"=15, "RS Stream"=3, "RS Format"=5, "index"=0, "width"=480, "height"=270, "ppx"=237.96481, "ppy"=139.0124, "fx"=357.2274, "fy"=357.2274, "model"=4}, {"ID"=41, "Profile"=521331352, "fps"=6, "RS Stream"=3, "RS Format"=14, "index"=0, "width"=480, "height"=270, "ppx"=237.96481, "ppy"=139.0124, "fx"=357.2274, "fy"=357.2274, "model"=4}, {"ID"=41, "Profile"=521324696, "fps"=6, "RS Stream"=3, "RS Format"=10, "index"=0, "width"=480, "height"=270, "ppx"=0.0, "ppy"=0.0, "fx"=0.0, "fy"=0.0, "model"=0}, {"ID"=42, "Profile"=521602488, "fps"=6, "RS Stream"=3, "RS Format"=9, "index"=2, "width"=480, "height"=270, "ppx"=237.96481, "ppy"=139.0124, "fx"=357.2274, "fy"=357.2274, "model"=4}, {"ID"=41, "Profile"=521314968, "fps"=6, "RS Stream"=3, "RS Format"=9, "index"=1, "width"=480, "height"=270, "ppx"=237.96481, "ppy"=139.0124, "fx"=357.2274, "fy"=357.2274, "model"=4}, {"ID"=41, "Profile"=521330072, "fps"=6, "RS Stream"=3, "RS Format"=8, "index"=0, "width"=480, "height"=270, "ppx"=237.96481, "ppy"=139.0124, "fx"=357.2274, "fy"=357.2274, "model"=4}, {"ID"=41, "Profile"=521326488, "fps"=6, "RS Stream"=3, "RS Format"=7, "index"=0, "width"=480, "height"=270, "ppx"=237.96481, "ppy"=139.0124, "fx"=357.2274, "fy"=357.2274, "model"=4}, {"ID"=41, "Profile"=521329304, "fps"=6, "RS Stream"=3, "RS Format"=6, "index"=0, "width"=480, "height"=270, "ppx"=237.96481, "ppy"=139.0124, "fx"=357.2274, "fy"=357.2274, "model"=4}, {"ID"=41, "Profile"=521329048, "fps"=6, "RS Stream"=3, "RS Format"=5, "index"=0, "width"=480, "height"=270, "ppx"=237.96481, "ppy"=139.0124, "fx"=357.2274, "fy"=357.2274, "model"=4}, {"ID"=41, "Profile"=521307032, "fps"=90, "RS Stream"=3, "RS Format"=14, "index"=0, "width"=424, "height"=240, "ppx"=210.19093, "ppy"=123.56658, "fx"=317.53546, "fy"=317.53546, "model"=4}, {"ID"=41, "Profile"=521322136, "fps"=90, "RS Stream"=3, "RS Format"=10, "index"=0, "width"=424, "height"=240, "ppx"=0.0, "ppy"=0.0, "fx"=0.0, "fy"=0.0, "model"=0}, {"ID"=42, "Profile"=521601976, "fps"=90, "RS Stream"=3, "RS Format"=9, "index"=2, "width"=424, "height"=240, "ppx"=210.19093, "ppy"=123.56658, "fx"=317.53546, "fy"=317.53546, "model"=4}, {"ID"=41, "Profile"=521315736, "fps"=90, "RS Stream"=3, "RS Format"=9, "index"=1, "width"=424, "height"=240, "ppx"=210.19093, "ppy"=123.56658, "fx"=317.53546, "fy"=317.53546, "model"=4}, {"ID"=41, "Profile"=521338776, "fps"=90, "RS Stream"=3, "RS Format"=8, "index"=0, "width"=424, "height"=240, "ppx"=210.19093, "ppy"=123.56658, "fx"=317.53546, "fy"=317.53546, "model"=4}, {"ID"=41, "Profile"=521307288, "fps"=90, "RS Stream"=3, "RS Format"=7, "index"=0, "width"=424, "height"=240, "ppx"=210.19093, "ppy"=123.56658, "fx"=317.53546, "fy"=317.53546, "model"=4}, {"ID"=41, "Profile"=521307544, "fps"=90, "RS Stream"=3, "RS Format"=6, "index"=0, "width"=424, "height"=240, "ppx"=210.19093, "ppy"=123.56658, "fx"=317.53546, "fy"=317.53546, "model"=4}, {"ID"=41, "Profile"=521321624, "fps"=90, "RS Stream"=3, "RS Format"=5, "index"=0, "width"=424, "height"=240, "ppx"=210.19093, "ppy"=123.56658, "fx"=317.53546, "fy"=317.53546, "model"=4}, {"ID"=41, "Profile"=521323928, "fps"=60, "RS Stream"=3, "RS Format"=14, "index"=0, "width"=424, "height"=240, "ppx"=210.19093, "ppy"=123.56658, "fx"=317.53546, "fy"=317.53546, "model"=4}, {"ID"=41, "Profile"=521339032, "fps"=60, "RS Stream"=3, "RS Format"=10, "index"=0, "width"=424, "height"=240, "ppx"=0.0, "ppy"=0.0, "fx"=0.0, "fy"=0.0, "model"=0}, {"ID"=42, "Profile"=521614008, "fps"=60, "RS Stream"=3, "RS Format"=9, "index"=2, "width"=424, "height"=240, "ppx"=210.19093, "ppy"=123.56658, "fx"=317.53546, "fy"=317.53546, "model"=4}, {"ID"=41, "Profile"=521313688, "fps"=60, "RS Stream"=3, "RS Format"=9, "index"=1, "width"=424, "height"=240, "ppx"=210.19093, "ppy"=123.56658, "fx"=317.53546, "fy"=317.53546, "model"=4}, {"ID"=41, "Profile"=521335192, "fps"=60, "RS Stream"=3, "RS Format"=8, "index"=0, "width"=424, "height"=240, "ppx"=210.19093, "ppy"=123.56658, "fx"=317.53546, "fy"=317.53546, "model"=4}, {"ID"=41, "Profile"=521337240, "fps"=60, "RS Stream"=3, "RS Format"=7, "index"=0, "width"=424, "height"=240, "ppx"=210.19093, "ppy"=123.56658, "fx"=317.53546, "fy"=317.53546, "model"=4}, {"ID"=41, "Profile"=521334680, "fps"=60, "RS Stream"=3, "RS Format"=6, "index"=0, "width"=424, "height"=240, "ppx"=210.19093, "ppy"=123.56658, "fx"=317.53546, "fy"=317.53546, "model"=4}, {"ID"=41, "Profile"=521334936, "fps"=60, "RS Stream"=3, "RS Format"=5, "index"=0, "width"=424, "height"=240, "ppx"=210.19093, "ppy"=123.56658, "fx"=317.53546, "fy"=317.53546, "model"=4}, {"ID"=41, "Profile"=521324952, "fps"=30, "RS Stream"=3, "RS Format"=14, "index"=0, "width"=424, "height"=240, "ppx"=210.19093, "ppy"=123.56658, "fx"=317.53546, "fy"=317.53546, "model"=4}, {"ID"=41, "Profile"=521335448, "fps"=30, "RS Stream"=3, "RS Format"=10, "index"=0, "width"=424, "height"=240, "ppx"=0.0, "ppy"=0.0, "fx"=0.0, "fy"=0.0, "model"=0}, {"ID"=42, "Profile"=521614264, "fps"=30, "RS Stream"=3, "RS Format"=9, "index"=2, "width"=424, "height"=240, "ppx"=210.19093, "ppy"=123.56658, "fx"=317.53546, "fy"=317.53546, "model"=4}, {"ID"=41, "Profile"=521314712, "fps"=30, "RS Stream"=3, "RS Format"=9, "index"=1, "width"=424, "height"=240, "ppx"=210.19093, "ppy"=123.56658, "fx"=317.53546, "fy"=317.53546, "model"=4}, {"ID"=41, "Profile"=521335704, "fps"=30, "RS Stream"=3, "RS Format"=8, "index"=0, "width"=424, "height"=240, "ppx"=210.19093, "ppy"=123.56658, "fx"=317.53546, "fy"=317.53546, "model"=4}, {"ID"=41, "Profile"=521327000, "fps"=30, "RS Stream"=3, "RS Format"=7, "index"=0, "width"=424, "height"=240, "ppx"=210.19093, "ppy"=123.56658, "fx"=317.53546, "fy"=317.53546, "model"=4}, {"ID"=41, "Profile"=521333656, "fps"=30, "RS Stream"=3, "RS Format"=6, "index"=0, "width"=424, "height"=240, "ppx"=210.19093, "ppy"=123.56658, "fx"=317.53546, "fy"=317.53546, "model"=4}, {"ID"=41, "Profile"=521336216, "fps"=30, "RS Stream"=3, "RS Format"=5, "index"=0, "width"=424, "height"=240, "ppx"=210.19093, "ppy"=123.56658, "fx"=317.53546, "fy"=317.53546, "model"=4}, {"ID"=41, "Profile"=521332376, "fps"=15, "RS Stream"=3, "RS Format"=14, "index"=0, "width"=424, "height"=240, "ppx"=210.19093, "ppy"=123.56658, "fx"=317.53546, "fy"=317.53546, "model"=4}, {"ID"=41, "Profile"=521339288, "fps"=15, "RS Stream"=3, "RS Format"=10, "index"=0, "width"=424, "height"=240, "ppx"=0.0, "ppy"=0.0, "fx"=0.0, "fy"=0.0, "model"=0}, {"ID"=42, "Profile"=521611192, "fps"=15, "RS Stream"=3, "RS Format"=9, "index"=2, "width"=424, "height"=240, "ppx"=210.19093, "ppy"=123.56658, "fx"=317.53546, "fy"=317.53546, "model"=4}, {"ID"=41, "Profile"=521310104, "fps"=15, "RS Stream"=3, "RS Format"=9, "index"=1, "width"=424, "height"=240, "ppx"=210.19093, "ppy"=123.56658, "fx"=317.53546, "fy"=317.53546, "model"=4}, {"ID"=41, "Profile"=521325208, "fps"=15, "RS Stream"=3, "RS Format"=8, "index"=0, "width"=424, "height"=240, "ppx"=210.19093, "ppy"=123.56658, "fx"=317.53546, "fy"=317.53546, "model"=4}, {"ID"=41, "Profile"=521329560, "fps"=15, "RS Stream"=3, "RS Format"=7, "index"=0, "width"=424, "height"=240, "ppx"=210.19093, "ppy"=123.56658, "fx"=317.53546, "fy"=317.53546, "model"=4}, {"ID"=41, "Profile"=521338008, "fps"=15, "RS Stream"=3, "RS Format"=6, "index"=0, "width"=424, "height"=240, "ppx"=210.19093, "ppy"=123.56658, "fx"=317.53546, "fy"=317.53546, "model"=4}, {"ID"=41, "Profile"=521335960, "fps"=15, "RS Stream"=3, "RS Format"=5, "index"=0, "width"=424, "height"=240, "ppx"=210.19093, "ppy"=123.56658, "fx"=317.53546, "fy"=317.53546, "model"=4}, {"ID"=41, "Profile"=521333400, "fps"=6, "RS Stream"=3, "RS Format"=14, "index"=0, "width"=424, "height"=240, "ppx"=210.19093, "ppy"=123.56658, "fx"=317.53546, "fy"=317.53546, "model"=4}, {"ID"=41, "Profile"=521334168, "fps"=6, "RS Stream"=3, "RS Format"=10, "index"=0, "width"=424, "height"=240, "ppx"=0.0, "ppy"=0.0, "fx"=0.0, "fy"=0.0, "model"=0}, {"ID"=42, "Profile"=521602232, "fps"=6, "RS Stream"=3, "RS Format"=9, "index"=2, "width"=424, "height"=240, "ppx"=210.19093, "ppy"=123.56658, "fx"=317.53546, "fy"=317.53546, "model"=4}, {"ID"=41, "Profile"=521311384, "fps"=6, "RS Stream"=3, "RS Format"=9, "index"=1, "width"=424, "height"=240, "ppx"=210.19093, "ppy"=123.56658, "fx"=317.53546, "fy"=317.53546, "model"=4}, {"ID"=41, "Profile"=521334424, "fps"=6, "RS Stream"=3, "RS Format"=8, "index"=0, "width"=424, "height"=240, "ppx"=210.19093, "ppy"=123.56658, "fx"=317.53546, "fy"=317.53546, "model"=4}, {"ID"=41, "Profile"=521323160, "fps"=6, "RS Stream"=3, "RS Format"=7, "index"=0, "width"=424, "height"=240, "ppx"=210.19093, "ppy"=123.56658, "fx"=317.53546, "fy"=317.53546, "model"=4}, {"ID"=41, "Profile"=521327512, "fps"=6, "RS Stream"=3, "RS Format"=6, "index"=0, "width"=424, "height"=240, "ppx"=210.19093, "ppy"=123.56658, "fx"=317.53546, "fy"=317.53546, "model"=4}, {"ID"=41, "Profile"=521327256, "fps"=6, "RS Stream"=3, "RS Format"=5, "index"=0, "width"=424, "height"=240, "ppx"=210.19093, "ppy"=123.56658, "fx"=317.53546, "fy"=317.53546, "model"=4}, {"ID"=40, "Profile"=521312408, "fps"=30, "RS Stream"=1, "RS Format"=2, "index"=0, "width"=1280, "height"=720, "ppx"=634.5728, "ppy"=370.69974, "fx"=952.6064, "fy"=952.6064, "model"=4}, {"ID"=40, "Profile"=521319832, "fps"=30, "RS Stream"=1, "RS Format"=1, "index"=0, "width"=1280, "height"=720, "ppx"=634.5728, "ppy"=370.69974, "fx"=952.6064, "fy"=952.6064, "model"=4}, {"ID"=40, "Profile"=521309336, "fps"=15, "RS Stream"=1, "RS Format"=2, "index"=0, "width"=1280, "height"=720, "ppx"=634.5728, "ppy"=370.69974, "fx"=952.6064, "fy"=952.6064, "model"=4}, {"ID"=40, "Profile"=521316248, "fps"=15, "RS Stream"=1, "RS Format"=1, "index"=0, "width"=1280, "height"=720, "ppx"=634.5728, "ppy"=370.69974, "fx"=952.6064, "fy"=952.6064, "model"=4}, {"ID"=40, "Profile"=521309080, "fps"=6, "RS Stream"=1, "RS Format"=2, "index"=0, "width"=1280, "height"=720, "ppx"=634.5728, "ppy"=370.69974, "fx"=952.6064, "fy"=952.6064, "model"=4}, {"ID"=40, "Profile"=521315224, "fps"=6, "RS Stream"=1, "RS Format"=1, "index"=0, "width"=1280, "height"=720, "ppx"=634.5728, "ppy"=370.69974, "fx"=952.6064, "fy"=952.6064, "model"=4}, {"ID"=40, "Profile"=521317784, "fps"=90, "RS Stream"=1, "RS Format"=2, "index"=0, "width"=848, "height"=480, "ppx"=420.38187, "ppy"=247.13316, "fx"=635.0709, "fy"=635.0709, "model"=4}, {"ID"=40, "Profile"=521322392, "fps"=90, "RS Stream"=1, "RS Format"=1, "index"=0, "width"=848, "height"=480, "ppx"=420.38187, "ppy"=247.13316, "fx"=635.0709, "fy"=635.0709, "model"=4}, {"ID"=40, "Profile"=521321880, "fps"=60, "RS Stream"=1, "RS Format"=2, "index"=0, "width"=848, "height"=480, "ppx"=420.38187, "ppy"=247.13316, "fx"=635.0709, "fy"=635.0709, "model"=4}, {"ID"=40, "Profile"=521318040, "fps"=60, "RS Stream"=1, "RS Format"=1, "index"=0, "width"=848, "height"=480, "ppx"=420.38187, "ppy"=247.13316, "fx"=635.0709, "fy"=635.0709, "model"=4}, {"ID"=40, "Profile"=521312920, "fps"=30, "RS Stream"=1, "RS Format"=2, "index"=0, "width"=848, "height"=480, "ppx"=420.38187, "ppy"=247.13316, "fx"=635.0709, "fy"=635.0709, "model"=4}, {"ID"=40, "Profile"=521320856, "fps"=30, "RS Stream"=1, "RS Format"=1, "index"=0, "width"=848, "height"=480, "ppx"=420.38187, "ppy"=247.13316, "fx"=635.0709, "fy"=635.0709, "model"=4}, {"ID"=40, "Profile"=521319576, "fps"=15, "RS Stream"=1, "RS Format"=2, "index"=0, "width"=848, "height"=480, "ppx"=420.38187, "ppy"=247.13316, "fx"=635.0709, "fy"=635.0709, "model"=4}, {"ID"=40, "Profile"=521308056, "fps"=15, "RS Stream"=1, "RS Format"=1, "index"=0, "width"=848, "height"=480, "ppx"=420.38187, "ppy"=247.13316, "fx"=635.0709, "fy"=635.0709, "model"=4}, {"ID"=40, "Profile"=521312664, "fps"=6, "RS Stream"=1, "RS Format"=2, "index"=0, "width"=848, "height"=480, "ppx"=420.38187, "ppy"=247.13316, "fx"=635.0709, "fy"=635.0709, "model"=4}, {"ID"=40, "Profile"=521308824, "fps"=6, "RS Stream"=1, "RS Format"=1, "index"=0, "width"=848, "height"=480, "ppx"=420.38187, "ppy"=247.13316, "fx"=635.0709, "fy"=635.0709, "model"=4}, {"ID"=40, "Profile"=521308568, "fps"=90, "RS Stream"=1, "RS Format"=2, "index"=0, "width"=640, "height"=480, "ppx"=316.38187, "ppy"=247.13316, "fx"=635.0709, "fy"=635.0709, "model"=4}, {"ID"=40, "Profile"=521313432, "fps"=90, "RS Stream"=1, "RS Format"=1, "index"=0, "width"=640, "height"=480, "ppx"=316.38187, "ppy"=247.13316, "fx"=635.0709, "fy"=635.0709, "model"=4}, {"ID"=40, "Profile"=521315480, "fps"=60, "RS Stream"=1, "RS Format"=2, "index"=0, "width"=640, "height"=480, "ppx"=316.38187, "ppy"=247.13316, "fx"=635.0709, "fy"=635.0709, "model"=4}, {"ID"=40, "Profile"=521318552, "fps"=60, "RS Stream"=1, "RS Format"=1, "index"=0, "width"=640, "height"=480, "ppx"=316.38187, "ppy"=247.13316, "fx"=635.0709, "fy"=635.0709, "model"=4}, {"ID"=40, "Profile"=521311128, "fps"=30, "RS Stream"=1, "RS Format"=2, "index"=0, "width"=640, "height"=480, "ppx"=316.38187, "ppy"=247.13316, "fx"=635.0709, "fy"=635.0709, "model"=4}, {"ID"=40, "Profile"=521309848, "fps"=30, "RS Stream"=1, "RS Format"=1, "index"=0, "width"=640, "height"=480, "ppx"=316.38187, "ppy"=247.13316, "fx"=635.0709, "fy"=635.0709, "model"=4}, {"ID"=40, "Profile"=521317528, "fps"=15, "RS Stream"=1, "RS Format"=2, "index"=0, "width"=640, "height"=480, "ppx"=316.38187, "ppy"=247.13316, "fx"=635.0709, "fy"=635.0709, "model"=4}, {"ID"=40, "Profile"=521316760, "fps"=15, "RS Stream"=1, "RS Format"=1, "index"=0, "width"=640, "height"=480, "ppx"=316.38187, "ppy"=247.13316, "fx"=635.0709, "fy"=635.0709, "model"=4}, {"ID"=40, "Profile"=521311896, "fps"=6, "RS Stream"=1, "RS Format"=2, "index"=0, "width"=640, "height"=480, "ppx"=316.38187, "ppy"=247.13316, "fx"=635.0709, "fy"=635.0709, "model"=4}, {"ID"=40, "Profile"=521307800, "fps"=6, "RS Stream"=1, "RS Format"=1, "index"=0, "width"=640, "height"=480, "ppx"=316.38187, "ppy"=247.13316, "fx"=635.0709, "fy"=635.0709, "model"=4}, {"ID"=40, "Profile"=521290648, "fps"=90, "RS Stream"=1, "RS Format"=2, "index"=0, "width"=640, "height"=360, "ppx"=317.2864, "ppy"=185.34987, "fx"=476.3032, "fy"=476.3032, "model"=4}, {"ID"=40, "Profile"=521306520, "fps"=90, "RS Stream"=1, "RS Format"=1, "index"=0, "width"=640, "height"=360, "ppx"=317.2864, "ppy"=185.34987, "fx"=476.3032, "fy"=476.3032, "model"=4}, {"ID"=40, "Profile"=521293208, "fps"=60, "RS Stream"=1, "RS Format"=2, "index"=0, "width"=640, "height"=360, "ppx"=317.2864, "ppy"=185.34987, "fx"=476.3032, "fy"=476.3032, "model"=4}, {"ID"=40, "Profile"=521292952, "fps"=60, "RS Stream"=1, "RS Format"=1, "index"=0, "width"=640, "height"=360, "ppx"=317.2864, "ppy"=185.34987, "fx"=476.3032, "fy"=476.3032, "model"=4}, {"ID"=40, "Profile"=521294232, "fps"=30, "RS Stream"=1, "RS Format"=2, "index"=0, "width"=640, "height"=360, "ppx"=317.2864, "ppy"=185.34987, "fx"=476.3032, "fy"=476.3032, "model"=4}, {"ID"=40, "Profile"=521293720, "fps"=30, "RS Stream"=1, "RS Format"=1, "index"=0, "width"=640, "height"=360, "ppx"=317.2864, "ppy"=185.34987, "fx"=476.3032, "fy"=476.3032, "model"=4}, {"ID"=40, "Profile"=521317016, "fps"=15, "RS Stream"=1, "RS Format"=2, "index"=0, "width"=640, "height"=360, "ppx"=317.2864, "ppy"=185.34987, "fx"=476.3032, "fy"=476.3032, "model"=4}, {"ID"=40, "Profile"=521308312, "fps"=15, "RS Stream"=1, "RS Format"=1, "index"=0, "width"=640, "height"=360, "ppx"=317.2864, "ppy"=185.34987, "fx"=476.3032, "fy"=476.3032, "model"=4}, {"ID"=40, "Profile"=521311640, "fps"=6, "RS Stream"=1, "RS Format"=2, "index"=0, "width"=640, "height"=360, "ppx"=317.2864, "ppy"=185.34987, "fx"=476.3032, "fy"=476.3032, "model"=4}, {"ID"=40, "Profile"=521313944, "fps"=6, "RS Stream"=1, "RS Format"=1, "index"=0, "width"=640, "height"=360, "ppx"=317.2864, "ppy"=185.34987, "fx"=476.3032, "fy"=476.3032, "model"=4}, {"ID"=40, "Profile"=521293464, "fps"=90, "RS Stream"=1, "RS Format"=2, "index"=0, "width"=480, "height"=270, "ppx"=237.96481, "ppy"=139.0124, "fx"=357.2274, "fy"=357.2274, "model"=4}, {"ID"=40, "Profile"=521297560, "fps"=90, "RS Stream"=1, "RS Format"=1, "index"=0, "width"=480, "height"=270, "ppx"=237.96481, "ppy"=139.0124, "fx"=357.2274, "fy"=357.2274, "model"=4}, {"ID"=40, "Profile"=521302680, "fps"=60, "RS Stream"=1, "RS Format"=2, "index"=0, "width"=480, "height"=270, "ppx"=237.96481, "ppy"=139.0124, "fx"=357.2274, "fy"=357.2274, "model"=4}, {"ID"=40, "Profile"=521300376, "fps"=60, "RS Stream"=1, "RS Format"=1, "index"=0, "width"=480, "height"=270, "ppx"=237.96481, "ppy"=139.0124, "fx"=357.2274, "fy"=357.2274, "model"=4}, {"ID"=40, "Profile"=521302936, "fps"=30, "RS Stream"=1, "RS Format"=2, "index"=0, "width"=480, "height"=270, "ppx"=237.96481, "ppy"=139.0124, "fx"=357.2274, "fy"=357.2274, "model"=4}, {"ID"=40, "Profile"=521301144, "fps"=30, "RS Stream"=1, "RS Format"=1, "index"=0, "width"=480, "height"=270, "ppx"=237.96481, "ppy"=139.0124, "fx"=357.2274, "fy"=357.2274, "model"=4}, {"ID"=40, "Profile"=521303192, "fps"=15, "RS Stream"=1, "RS Format"=2, "index"=0, "width"=480, "height"=270, "ppx"=237.96481, "ppy"=139.0124, "fx"=357.2274, "fy"=357.2274, "model"=4}, {"ID"=40, "Profile"=521304984, "fps"=15, "RS Stream"=1, "RS Format"=1, "index"=0, "width"=480, "height"=270, "ppx"=237.96481, "ppy"=139.0124, "fx"=357.2274, "fy"=357.2274, "model"=4}, {"ID"=40, "Profile"=521304216, "fps"=6, "RS Stream"=1, "RS Format"=2, "index"=0, "width"=480, "height"=270, "ppx"=237.96481, "ppy"=139.0124, "fx"=357.2274, "fy"=357.2274, "model"=4}, {"ID"=40, "Profile"=521303704, "fps"=6, "RS Stream"=1, "RS Format"=1, "index"=0, "width"=480, "height"=270, "ppx"=237.96481, "ppy"=139.0124, "fx"=357.2274, "fy"=357.2274, "model"=4}, {"ID"=40, "Profile"=521306264, "fps"=90, "RS Stream"=1, "RS Format"=2, "index"=0, "width"=424, "height"=240, "ppx"=210.19093, "ppy"=123.56658, "fx"=317.53546, "fy"=317.53546, "model"=4}, {"ID"=40, "Profile"=521301912, "fps"=90, "RS Stream"=1, "RS Format"=1, "index"=0, "width"=424, "height"=240, "ppx"=210.19093, "ppy"=123.56658, "fx"=317.53546, "fy"=317.53546, "model"=4}, {"ID"=40, "Profile"=521292184, "fps"=60, "RS Stream"=1, "RS Format"=2, "index"=0, "width"=424, "height"=240, "ppx"=210.19093, "ppy"=123.56658, "fx"=317.53546, "fy"=317.53546, "model"=4}, {"ID"=40, "Profile"=521291928, "fps"=60, "RS Stream"=1, "RS Format"=1, "index"=0, "width"=424, "height"=240, "ppx"=210.19093, "ppy"=123.56658, "fx"=317.53546, "fy"=317.53546, "model"=4}, {"ID"=40, "Profile"=521296792, "fps"=30, "RS Stream"=1, "RS Format"=2, "index"=0, "width"=424, "height"=240, "ppx"=210.19093, "ppy"=123.56658, "fx"=317.53546, "fy"=317.53546, "model"=4}, {"ID"=40, "Profile"=521300120, "fps"=30, "RS Stream"=1, "RS Format"=1, "index"=0, "width"=424, "height"=240, "ppx"=210.19093, "ppy"=123.56658, "fx"=317.53546, "fy"=317.53546, "model"=4}, {"ID"=40, "Profile"=521300632, "fps"=15, "RS Stream"=1, "RS Format"=2, "index"=0, "width"=424, "height"=240, "ppx"=210.19093, "ppy"=123.56658, "fx"=317.53546, "fy"=317.53546, "model"=4}, {"ID"=40, "Profile"=521302424, "fps"=15, "RS Stream"=1, "RS Format"=1, "index"=0, "width"=424, "height"=240, "ppx"=210.19093, "ppy"=123.56658, "fx"=317.53546, "fy"=317.53546, "model"=4}, {"ID"=40, "Profile"=521300888, "fps"=6, "RS Stream"=1, "RS Format"=2, "index"=0, "width"=424, "height"=240, "ppx"=210.19093, "ppy"=123.56658, "fx"=317.53546, "fy"=317.53546, "model"=4}, {"ID"=40, "Profile"=521292696, "fps"=6, "RS Stream"=1, "RS Format"=1, "index"=0, "width"=424, "height"=240, "ppx"=210.19093, "ppy"=123.56658, "fx"=317.53546, "fy"=317.53546, "model"=4}] {"model" items=["RS_DISTORTION_NONE", "RS_DISTORTION_MODIFIED_BROWN_CONRADY", "RS_DISTORTION_INVERSE_BROWN_CONRADY", "RS_DISTORTION_FTHETA", "RS_DISTORTION_BROWN_CONRADY", "RS_DISTORTION_COUNT"]; "RS Format" items=["    RS2_FORMAT_ANY             , /**< When passed to enable stream, librealsense will try to provide best suited format */", "    RS2_FORMAT_Z16             , /**< 16-bit linear depth values. The depth is meters is equal to depth scale * pixel value. */", "    RS2_FORMAT_DISPARITY16     , /**< 16-bit linear disparity values. The depth in meters is equal to depth scale / pixel value. */", "    RS2_FORMAT_XYZ32F          , /**< 32-bit floating point 3D coordinates. */", "    RS2_FORMAT_YUYV            , /**< Standard YUV pixel format as described in https://en.wikipedia.org/wiki/YUV */", "    RS2_FORMAT_RGB8            , /**< 8-bit red, green and blue channels */", "    RS2_FORMAT_BGR8            , /**< 8-bit blue, green, and red channels -- suitable for OpenCV */", "    RS2_FORMAT_RGBA8           , /**< 8-bit red, green and blue channels + constant alpha channel equal to FF */", "    RS2_FORMAT_BGRA8           , /**< 8-bit blue, green, and red channels + constant alpha channel equal to FF */", "    RS2_FORMAT_Y8              , /**< 8-bit per-pixel grayscale image */", "    RS2_FORMAT_Y16             , /**< 16-bit per-pixel grayscale image */", "    RS2_FORMAT_RAW10           , /**< Four 10-bit luminance values encoded into a 5-byte macropixel */", "    RS2_FORMAT_RAW16           , /**< 16-bit raw image */", "    RS2_FORMAT_RAW8            , /**< 8-bit raw image */", "    RS2_FORMAT_UYVY            , /**< Similar to the standard YUYV pixel format, but packed in a different order */", "    RS2_FORMAT_MOTION_RAW      , /**< Raw data from the motion sensor */", "    RS2_FORMAT_MOTION_XYZ32F   , /**< Motion data packed as 3 32-bit float values, for X, Y, and Z axis */", "    RS2_FORMAT_GPIO_RAW        , /**< Raw data from the external sensors hooked to one of the GPIO's */", "    RS2_FORMAT_COUNT             /**< Number of enumeration values. Not a valid input: intended to be used in for-loops. */"]; "RS Stream" items=["    RS2_STREAM_ANY,", "    RS2_STREAM_DEPTH                            , /**< Native stream of depth data produced by RealSense device */", "    RS2_STREAM_COLOR                            , /**< Native stream of color data captured by RealSense device */", "    RS2_STREAM_INFRARED                         , /**< Native stream of infrared data captured by RealSense device */", "    RS2_STREAM_FISHEYE                          , /**< Native stream of fish-eye (wide) data captured from the dedicate motion camera */", "    RS2_STREAM_GYRO                             , /**< Native stream of gyroscope motion data produced by RealSense device */", "    RS2_STREAM_ACCEL                            , /**< Native stream of accelerometer motion data produced by RealSense device */", "    RS2_STREAM_GPIO                             , /**< Signals from external device connected through GPIO */", "    RS2_STREAM_COUNT"]}) -> (1 "IR Left Array":string[](array[string])=["424 x 240 @6fps", "424 x 240 @15fps", "424 x 240 @30fps", "424 x 240 @60fps", "424 x 240 @90fps", "480 x 270 @6fps", "480 x 270 @15fps", "480 x 270 @30fps", "480 x 270 @60fps", "480 x 270 @90fps", "640 x 360 @6fps", "640 x 360 @15fps", "640 x 360 @30fps", "640 x 360 @60fps", "640 x 360 @90fps", "640 x 480 @6fps", "640 x 480 @15fps", "640 x 480 @30fps", "640 x 480 @60fps", "640 x 480 @90fps", "848 x 480 @6fps", "848 x 480 @15fps", "848 x 480 @30fps", "848 x 480 @60fps", "848 x 480 @90fps", "1280 x 720 @6fps", "1280 x 720 @15fps", "1280 x 720 @30fps", "1920 x 1080 @15fps", "1920 x 1080 @25fps"], 2 "Unrectified R IR":string[](array[string])=["424 x 240 @6fps", "424 x 240 @15fps", "424 x 240 @30fps", "424 x 240 @60fps", "424 x 240 @90fps", "480 x 270 @6fps", "480 x 270 @15fps", "480 x 270 @30fps", "480 x 270 @60fps", "480 x 270 @90fps", "640 x 360 @6fps", "640 x 360 @15fps", "640 x 360 @30fps", "640 x 360 @60fps", "640 x 360 @90fps", "640 x 480 @6fps", "640 x 480 @15fps", "640 x 480 @30fps", "640 x 480 @60fps", "640 x 480 @90fps", "848 x 480 @6fps", "848 x 480 @15fps", "848 x 480 @30fps", "848 x 480 @60fps", "848 x 480 @90fps", "1280 x 720 @6fps", "1280 x 720 @15fps", "1280 x 720 @30fps"], 3 "IR left":T1(array[cluster])=[{"width"=424, "height"=240, "fps"=6, "Profile"=521311384, "ppx"=210.19093, "ppy"=123.56658, "fx"=317.53546, "fy"=317.53546, "model"=4}, {"width"=424, "height"=240, "fps"=15, "Profile"=521310104, "ppx"=210.19093, "ppy"=123.56658, "fx"=317.53546, "fy"=317.53546, "model"=4}, {"width"=424, "height"=240, "fps"=30, "Profile"=521314712, "ppx"=210.19093, "ppy"=123.56658, "fx"=317.53546, "fy"=317.53546, "model"=4}, {"width"=424, "height"=240, "fps"=60, "Profile"=521313688, "ppx"=210.19093, "ppy"=123.56658, "fx"=317.53546, "fy"=317.53546, "model"=4}, {"width"=424, "height"=240, "fps"=90, "Profile"=521315736, "ppx"=210.19093, "ppy"=123.56658, "fx"=317.53546, "fy"=317.53546, "model"=4}, {"width"=480, "height"=270, "fps"=6, "Profile"=521314968, "ppx"=237.96481, "ppy"=139.0124, "fx"=357.2274, "fy"=357.2274, "model"=4}, {"width"=480, "height"=270, "fps"=15, "Profile"=521318808, "ppx"=237.96481, "ppy"=139.0124, "fx"=357.2274, "fy"=357.2274, "model"=4}, {"width"=480, "height"=270, "fps"=30, "Profile"=521316504, "ppx"=237.96481, "ppy"=139.0124, "fx"=357.2274, "fy"=357.2274, "model"=4}, {"width"=480, "height"=270, "fps"=60, "Profile"=521322904, "ppx"=237.96481, "ppy"=139.0124, "fx"=357.2274, "fy"=357.2274, "model"=4}, {"width"=480, "height"=270, "fps"=90, "Profile"=521312152, "ppx"=237.96481, "ppy"=139.0124, "fx"=357.2274, "fy"=357.2274, "model"=4}, {"width"=640, "height"=360, "fps"=6, "Profile"=521314200, "ppx"=317.2864, "ppy"=185.34987, "fx"=476.3032, "fy"=476.3032, "model"=4}, {"width"=640, "height"=360, "fps"=15, "Profile"=521319320, "ppx"=317.2864, "ppy"=185.34987, "fx"=476.3032, "fy"=476.3032, "model"=4}, {"width"=640, "height"=360, "fps"=30, "Profile"=521319064, "ppx"=317.2864, "ppy"=185.34987, "fx"=476.3032, "fy"=476.3032, "model"=4}, {"width"=640, "height"=360, "fps"=60, "Profile"=521321112, "ppx"=317.2864, "ppy"=185.34987, "fx"=476.3032, "fy"=476.3032, "model"=4}, {"width"=640, "height"=360, "fps"=90, "Profile"=521318296, "ppx"=317.2864, "ppy"=185.34987, "fx"=476.3032, "fy"=476.3032, "model"=4}, {"width"=640, "height"=480, "fps"=6, "Profile"=521313176, "ppx"=316.38187, "ppy"=247.13316, "fx"=635.0709, "fy"=635.0709, "model"=4}, {"width"=640, "height"=480, "fps"=15, "Profile"=521321368, "ppx"=316.38187, "ppy"=247.13316, "fx"=635.0709, "fy"=635.0709, "model"=4}, {"width"=640, "height"=480, "fps"=30, "Profile"=521309592, "ppx"=316.38187, "ppy"=247.13316, "fx"=635.0709, "fy"=635.0709, "model"=4}, {"width"=640, "height"=480, "fps"=60, "Profile"=521320088, "ppx"=316.38187, "ppy"=247.13316, "fx"=635.0709, "fy"=635.0709, "model"=4}, {"width"=640, "height"=480, "fps"=90, "Profile"=521322648, "ppx"=316.38187, "ppy"=247.13316, "fx"=635.0709, "fy"=635.0709, "model"=4}, {"width"=848, "height"=480, "fps"=6, "Profile"=521315992, "ppx"=420.38187, "ppy"=247.13316, "fx"=635.0709, "fy"=635.0709, "model"=4}, {"width"=848, "height"=480, "fps"=15, "Profile"=521317272, "ppx"=420.38187, "ppy"=247.13316, "fx"=635.0709, "fy"=635.0709, "model"=4}, {"width"=848, "height"=480, "fps"=30, "Profile"=521310616, "ppx"=420.38187, "ppy"=247.13316, "fx"=635.0709, "fy"=635.0709, "model"=4}, {"width"=848, "height"=480, "fps"=60, "Profile"=521310360, "ppx"=420.38187, "ppy"=247.13316, "fx"=635.0709, "fy"=635.0709, "model"=4}, {"width"=848, "height"=480, "fps"=90, "Profile"=521306776, "ppx"=420.38187, "ppy"=247.13316, "fx"=635.0709, "fy"=635.0709, "model"=4}, {"width"=1280, "height"=720, "fps"=6, "Profile"=521320600, "ppx"=634.5728, "ppy"=370.69974, "fx"=952.6064, "fy"=952.6064, "model"=4}, {"width"=1280, "height"=720, "fps"=15, "Profile"=521310872, "ppx"=634.5728, "ppy"=370.69974, "fx"=952.6064, "fy"=952.6064, "model"=4}, {"width"=1280, "height"=720, "fps"=30, "Profile"=521320344, "ppx"=634.5728, "ppy"=370.69974, "fx"=952.6064, "fy"=952.6064, "model"=4}, {"width"=1920, "height"=1080, "fps"=15, "Profile"=521627576, "ppx"=951.85925, "ppy"=556.0496, "fx"=1428.9095, "fy"=1428.9095, "model"=4}, {"width"=1920, "height"=1080, "fps"=25, "Profile"=521617080, "ppx"=951.85925, "ppy"=556.0496, "fx"=1428.9095, "fy"=1428.9095, "model"=4}], 4 "Depth Stream":T1(array[cluster])=[{"width"=424, "height"=240, "fps"=6, "Profile"=521292696, "ppx"=210.19093, "ppy"=123.56658, "fx"=317.53546, "fy"=317.53546, "model"=4}, {"width"=424, "height"=240, "fps"=15, "Profile"=521302424, "ppx"=210.19093, "ppy"=123.56658, "fx"=317.53546, "fy"=317.53546, "model"=4}, {"width"=424, "height"=240, "fps"=30, "Profile"=521300120, "ppx"=210.19093, "ppy"=123.56658, "fx"=317.53546, "fy"=317.53546, "model"=4}, {"width"=424, "height"=240, "fps"=60, "Profile"=521291928, "ppx"=210.19093, "ppy"=123.56658, "fx"=317.53546, "fy"=317.53546, "model"=4}, {"width"=424, "height"=240, "fps"=90, "Profile"=521301912, "ppx"=210.19093, "ppy"=123.56658, "fx"=317.53546, "fy"=317.53546, "model"=4}, {"width"=480, "height"=270, "fps"=6, "Profile"=521303704, "ppx"=237.96481, "ppy"=139.0124, "fx"=357.2274, "fy"=357.2274, "model"=4}, {"width"=480, "height"=270, "fps"=15, "Profile"=521304984, "ppx"=237.96481, "ppy"=139.0124, "fx"=357.2274, "fy"=357.2274, "model"=4}, {"width"=480, "height"=270, "fps"=30, "Profile"=521301144, "ppx"=237.96481, "ppy"=139.0124, "fx"=357.2274, "fy"=357.2274, "model"=4}, {"width"=480, "height"=270, "fps"=60, "Profile"=521300376, "ppx"=237.96481, "ppy"=139.0124, "fx"=357.2274, "fy"=357.2274, "model"=4}, {"width"=480, "height"=270, "fps"=90, "Profile"=521297560, "ppx"=237.96481, "ppy"=139.0124, "fx"=357.2274, "fy"=357.2274, "model"=4}, {"width"=640, "height"=360, "fps"=6, "Profile"=521313944, "ppx"=317.2864, "ppy"=185.34987, "fx"=476.3032, "fy"=476.3032, "model"=4}, {"width"=640, "height"=360, "fps"=15, "Profile"=521308312, "ppx"=317.2864, "ppy"=185.34987, "fx"=476.3032, "fy"=476.3032, "model"=4}, {"width"=640, "height"=360, "fps"=30, "Profile"=521293720, "ppx"=317.2864, "ppy"=185.34987, "fx"=476.3032, "fy"=476.3032, "model"=4}, {"width"=640, "height"=360, "fps"=60, "Profile"=521292952, "ppx"=317.2864, "ppy"=185.34987, "fx"=476.3032, "fy"=476.3032, "model"=4}, {"width"=640, "height"=360, "fps"=90, "Profile"=521306520, "ppx"=317.2864, "ppy"=185.34987, "fx"=476.3032, "fy"=476.3032, "model"=4}, {"width"=640, "height"=480, "fps"=6, "Profile"=521307800, "ppx"=316.38187, "ppy"=247.13316, "fx"=635.0709, "fy"=635.0709, "model"=4}, {"width"=640, "height"=480, "fps"=15, "Profile"=521316760, "ppx"=316.38187, "ppy"=247.13316, "fx"=635.0709, "fy"=635.0709, "model"=4}, {"width"=640, "height"=480, "fps"=30, "Profile"=521309848, "ppx"=316.38187, "ppy"=247.13316, "fx"=635.0709, "fy"=635.0709, "model"=4}, {"width"=640, "height"=480, "fps"=60, "Profile"=521318552, "ppx"=316.38187, "ppy"=247.13316, "fx"=635.0709, "fy"=635.0709, "model"=4}, {"width"=640, "height"=480, "fps"=90, "Profile"=521313432, "ppx"=316.38187, "ppy"=247.13316, "fx"=635.0709, "fy"=635.0709, "model"=4}, {"width"=848, "height"=480, "fps"=6, "Profile"=521308824, "ppx"=420.38187, "ppy"=247.13316, "fx"=635.0709, "fy"=635.0709, "model"=4}, {"width"=848, "height"=480, "fps"=15, "Profile"=521308056, "ppx"=420.38187, "ppy"=247.13316, "fx"=635.0709, "fy"=635.0709, "model"=4}, {"width"=848, "height"=480, "fps"=30, "Profile"=521320856, "ppx"=420.38187, "ppy"=247.13316, "fx"=635.0709, "fy"=635.0709, "model"=4}, {"width"=848, "height"=480, "fps"=60, "Profile"=521318040, "ppx"=420.38187, "ppy"=247.13316, "fx"=635.0709, "fy"=635.0709, "model"=4}, {"width"=848, "height"=480, "fps"=90, "Profile"=521322392, "ppx"=420.38187, "ppy"=247.13316, "fx"=635.0709, "fy"=635.0709, "model"=4}, {"width"=1280, "height"=720, "fps"=6, "Profile"=521315224, "ppx"=634.5728, "ppy"=370.69974, "fx"=952.6064, "fy"=952.6064, "model"=4}, {"width"=1280, "height"=720, "fps"=15, "Profile"=521316248, "ppx"=634.5728, "ppy"=370.69974, "fx"=952.6064, "fy"=952.6064, "model"=4}, {"width"=1280, "height"=720, "fps"=30, "Profile"=521319832, "ppx"=634.5728, "ppy"=370.69974, "fx"=952.6064, "fy"=952.6064, "model"=4}], 5 "RGB ext.":T1(array[cluster])=[{"width"=424, "height"=240, "fps"=6, "Profile"=521292696, "ppx"=210.19093, "ppy"=123.56658, "fx"=317.53546, "fy"=317.53546, "model"=4}, {"width"=424, "height"=240, "fps"=15, "Profile"=521302424, "ppx"=210.19093, "ppy"=123.56658, "fx"=317.53546, "fy"=317.53546, "model"=4}, {"width"=424, "height"=240, "fps"=30, "Profile"=521300120, "ppx"=210.19093, "ppy"=123.56658, "fx"=317.53546, "fy"=317.53546, "model"=4}, {"width"=424, "height"=240, "fps"=60, "Profile"=521291928, "ppx"=210.19093, "ppy"=123.56658, "fx"=317.53546, "fy"=317.53546, "model"=4}, {"width"=424, "height"=240, "fps"=90, "Profile"=521301912, "ppx"=210.19093, "ppy"=123.56658, "fx"=317.53546, "fy"=317.53546, "model"=4}, {"width"=480, "height"=270, "fps"=6, "Profile"=521303704, "ppx"=237.96481, "ppy"=139.0124, "fx"=357.2274, "fy"=357.2274, "model"=4}, {"width"=480, "height"=270, "fps"=15, "Profile"=521304984, "ppx"=237.96481, "ppy"=139.0124, "fx"=357.2274, "fy"=357.2274, "model"=4}, {"width"=480, "height"=270, "fps"=30, "Profile"=521301144, "ppx"=237.96481, "ppy"=139.0124, "fx"=357.2274, "fy"=357.2274, "model"=4}, {"width"=480, "height"=270, "fps"=60, "Profile"=521300376, "ppx"=237.96481, "ppy"=139.0124, "fx"=357.2274, "fy"=357.2274, "model"=4}, {"width"=480, "height"=270, "fps"=90, "Profile"=521297560, "ppx"=237.96481, "ppy"=139.0124, "fx"=357.2274, "fy"=357.2274, "model"=4}, {"width"=640, "height"=360, "fps"=6, "Profile"=521313944, "ppx"=317.2864, "ppy"=185.34987, "fx"=476.3032, "fy"=476.3032, "model"=4}, {"width"=640, "height"=360, "fps"=15, "Profile"=521308312, "ppx"=317.2864, "ppy"=185.34987, "fx"=476.3032, "fy"=476.3032, "model"=4}, {"width"=640, "height"=360, "fps"=30, "Profile"=521293720, "ppx"=317.2864, "ppy"=185.34987, "fx"=476.3032, "fy"=476.3032, "model"=4}, {"width"=640, "height"=360, "fps"=60, "Profile"=521292952, "ppx"=317.2864, "ppy"=185.34987, "fx"=476.3032, "fy"=476.3032, "model"=4}, {"width"=640, "height"=360, "fps"=90, "Profile"=521306520, "ppx"=317.2864, "ppy"=185.34987, "fx"=476.3032, "fy"=476.3032, "model"=4}, {"width"=640, "height"=480, "fps"=6, "Profile"=521307800, "ppx"=316.38187, "ppy"=247.13316, "fx"=635.0709, "fy"=635.0709, "model"=4}, {"width"=640, "height"=480, "fps"=15, "Profile"=521316760, "ppx"=316.38187, "ppy"=247.13316, "fx"=635.0709, "fy"=635.0709, "model"=4}, {"width"=640, "height"=480, "fps"=30, "Profile"=521309848, "ppx"=316.38187, "ppy"=247.13316, "fx"=635.0709, "fy"=635.0709, "model"=4}, {"width"=640, "height"=480, "fps"=60, "Profile"=521318552, "ppx"=316.38187, "ppy"=247.13316, "fx"=635.0709, "fy"=635.0709, "model"=4}, {"width"=640, "height"=480, "fps"=90, "Profile"=521313432, "ppx"=316.38187, "ppy"=247.13316, "fx"=635.0709, "fy"=635.0709, "model"=4}, {"width"=848, "height"=480, "fps"=6, "Profile"=521308824, "ppx"=420.38187, "ppy"=247.13316, "fx"=635.0709, "fy"=635.0709, "model"=4}, {"width"=848, "height"=480, "fps"=15, "Profile"=521308056, "ppx"=420.38187, "ppy"=247.13316, "fx"=635.0709, "fy"=635.0709, "model"=4}, {"width"=848, "height"=480, "fps"=30, "Profile"=521320856, "ppx"=420.38187, "ppy"=247.13316, "fx"=635.0709, "fy"=635.0709, "model"=4}, {"width"=848, "height"=480, "fps"=60, "Profile"=521318040, "ppx"=420.38187, "ppy"=247.13316, "fx"=635.0709, "fy"=635.0709, "model"=4}, {"width"=848, "height"=480, "fps"=90, "Profile"=521322392, "ppx"=420.38187, "ppy"=247.13316, "fx"=635.0709, "fy"=635.0709, "model"=4}, {"width"=1280, "height"=720, "fps"=6, "Profile"=521315224, "ppx"=634.5728, "ppy"=370.69974, "fx"=952.6064, "fy"=952.6064, "model"=4}, {"width"=1280, "height"=720, "fps"=15, "Profile"=521316248, "ppx"=634.5728, "ppy"=370.69974, "fx"=952.6064, "fy"=952.6064, "model"=4}, {"width"=1280, "height"=720, "fps"=30, "Profile"=521319832, "ppx"=634.5728, "ppy"=370.69974, "fx"=952.6064, "fy"=952.6064, "model"=4}], 6 "Depth Stream strings":string[](array[string])=["424 x 240 @6fps", "424 x 240 @15fps", "424 x 240 @30fps", "424 x 240 @60fps", "424 x 240 @90fps", "480 x 270 @6fps", "480 x 270 @15fps", "480 x 270 @30fps", "480 x 270 @60fps", "480 x 270 @90fps", "640 x 360 @6fps", "640 x 360 @15fps", "640 x 360 @30fps", "640 x 360 @60fps", "640 x 360 @90fps", "640 x 480 @6fps", "640 x 480 @15fps", "640 x 480 @30fps", "640 x 480 @60fps", "640 x 480 @90fps", "848 x 480 @6fps", "848 x 480 @15fps", "848 x 480 @30fps", "848 x 480 @60fps", "848 x 480 @90fps", "1280 x 720 @6fps", "1280 x 720 @15fps", "1280 x 720 @30fps"], 7 "RGB ext.":string[](array[string])=["424 x 240 @6fps", "424 x 240 @15fps", "424 x 240 @30fps", "424 x 240 @60fps", "424 x 240 @90fps", "480 x 270 @6fps", "480 x 270 @15fps", "480 x 270 @30fps", "480 x 270 @60fps", "480 x 270 @90fps", "640 x 360 @6fps", "640 x 360 @15fps", "640 x 360 @30fps", "640 x 360 @60fps", "640 x 360 @90fps", "640 x 480 @6fps", "640 x 480 @15fps", "640 x 480 @30fps", "640 x 480 @60fps", "640 x 480 @90fps", "848 x 480 @6fps", "848 x 480 @15fps", "848 x 480 @30fps", "848 x 480 @60fps", "848 x 480 @90fps", "1280 x 720 @6fps", "1280 x 720 @15fps", "1280 x 720 @30fps"], 9 "Unrectified L IR":T1(array[cluster])=[{"width"=424, "height"=240, "fps"=6, "Profile"=521292696, "ppx"=210.19093, "ppy"=123.56658, "fx"=317.53546, "fy"=317.53546, "model"=4}, {"width"=424, "height"=240, "fps"=15, "Profile"=521302424, "ppx"=210.19093, "ppy"=123.56658, "fx"=317.53546, "fy"=317.53546, "model"=4}, {"width"=424, "height"=240, "fps"=30, "Profile"=521300120, "ppx"=210.19093, "ppy"=123.56658, "fx"=317.53546, "fy"=317.53546, "model"=4}, {"width"=424, "height"=240, "fps"=60, "Profile"=521291928, "ppx"=210.19093, "ppy"=123.56658, "fx"=317.53546, "fy"=317.53546, "model"=4}, {"width"=424, "height"=240, "fps"=90, "Profile"=521301912, "ppx"=210.19093, "ppy"=123.56658, "fx"=317.53546, "fy"=317.53546, "model"=4}, {"width"=480, "height"=270, "fps"=6, "Profile"=521303704, "ppx"=237.96481, "ppy"=139.0124, "fx"=357.2274, "fy"=357.2274, "model"=4}, {"width"=480, "height"=270, "fps"=15, "Profile"=521304984, "ppx"=237.96481, "ppy"=139.0124, "fx"=357.2274, "fy"=357.2274, "model"=4}, {"width"=480, "height"=270, "fps"=30, "Profile"=521301144, "ppx"=237.96481, "ppy"=139.0124, "fx"=357.2274, "fy"=357.2274, "model"=4}, {"width"=480, "height"=270, "fps"=60, "Profile"=521300376, "ppx"=237.96481, "ppy"=139.0124, "fx"=357.2274, "fy"=357.2274, "model"=4}, {"width"=480, "height"=270, "fps"=90, "Profile"=521297560, "ppx"=237.96481, "ppy"=139.0124, "fx"=357.2274, "fy"=357.2274, "model"=4}, {"width"=640, "height"=360, "fps"=6, "Profile"=521313944, "ppx"=317.2864, "ppy"=185.34987, "fx"=476.3032, "fy"=476.3032, "model"=4}, {"width"=640, "height"=360, "fps"=15, "Profile"=521308312, "ppx"=317.2864, "ppy"=185.34987, "fx"=476.3032, "fy"=476.3032, "model"=4}, {"width"=640, "height"=360, "fps"=30, "Profile"=521293720, "ppx"=317.2864, "ppy"=185.34987, "fx"=476.3032, "fy"=476.3032, "model"=4}, {"width"=640, "height"=360, "fps"=60, "Profile"=521292952, "ppx"=317.2864, "ppy"=185.34987, "fx"=476.3032, "fy"=476.3032, "model"=4}, {"width"=640, "height"=360, "fps"=90, "Profile"=521306520, "ppx"=317.2864, "ppy"=185.34987, "fx"=476.3032, "fy"=476.3032, "model"=4}, {"width"=640, "height"=480, "fps"=6, "Profile"=521307800, "ppx"=316.38187, "ppy"=247.13316, "fx"=635.0709, "fy"=635.0709, "model"=4}, {"width"=640, "height"=480, "fps"=15, "Profile"=521316760, "ppx"=316.38187, "ppy"=247.13316, "fx"=635.0709, "fy"=635.0709, "model"=4}, {"width"=640, "height"=480, "fps"=30, "Profile"=521309848, "ppx"=316.38187, "ppy"=247.13316, "fx"=635.0709, "fy"=635.0709, "model"=4}, {"width"=640, "height"=480, "fps"=60, "Profile"=521318552, "ppx"=316.38187, "ppy"=247.13316, "fx"=635.0709, "fy"=635.0709, "model"=4}, {"width"=640, "height"=480, "fps"=90, "Profile"=521313432, "ppx"=316.38187, "ppy"=247.13316, "fx"=635.0709, "fy"=635.0709, "model"=4}, {"width"=848, "height"=480, "fps"=6, "Profile"=521308824, "ppx"=420.38187, "ppy"=247.13316, "fx"=635.0709, "fy"=635.0709, "model"=4}, {"width"=848, "height"=480, "fps"=15, "Profile"=521308056, "ppx"=420.38187, "ppy"=247.13316, "fx"=635.0709, "fy"=635.0709, "model"=4}, {"width"=848, "height"=480, "fps"=30, "Profile"=521320856, "ppx"=420.38187, "ppy"=247.13316, "fx"=635.0709, "fy"=635.0709, "model"=4}, {"width"=848, "height"=480, "fps"=60, "Profile"=521318040, "ppx"=420.38187, "ppy"=247.13316, "fx"=635.0709, "fy"=635.0709, "model"=4}, {"width"=848, "height"=480, "fps"=90, "Profile"=521322392, "ppx"=420.38187, "ppy"=247.13316, "fx"=635.0709, "fy"=635.0709, "model"=4}, {"width"=1280, "height"=720, "fps"=6, "Profile"=521315224, "ppx"=634.5728, "ppy"=370.69974, "fx"=952.6064, "fy"=952.6064, "model"=4}, {"width"=1280, "height"=720, "fps"=15, "Profile"=521316248, "ppx"=634.5728, "ppy"=370.69974, "fx"=952.6064, "fy"=952.6064, "model"=4}, {"width"=1280, "height"=720, "fps"=30, "Profile"=521319832, "ppx"=634.5728, "ppy"=370.69974, "fx"=952.6064, "fy"=952.6064, "model"=4}], 10 "Color Left":T1(array[cluster])=[{"width"=424, "height"=240, "fps"=6, "Profile"=521327256, "ppx"=210.19093, "ppy"=123.56658, "fx"=317.53546, "fy"=317.53546, "model"=4}, {"width"=424, "height"=240, "fps"=15, "Profile"=521335960, "ppx"=210.19093, "ppy"=123.56658, "fx"=317.53546, "fy"=317.53546, "model"=4}, {"width"=424, "height"=240, "fps"=30, "Profile"=521336216, "ppx"=210.19093, "ppy"=123.56658, "fx"=317.53546, "fy"=317.53546, "model"=4}, {"width"=424, "height"=240, "fps"=60, "Profile"=521334936, "ppx"=210.19093, "ppy"=123.56658, "fx"=317.53546, "fy"=317.53546, "model"=4}, {"width"=424, "height"=240, "fps"=90, "Profile"=521321624, "ppx"=210.19093, "ppy"=123.56658, "fx"=317.53546, "fy"=317.53546, "model"=4}, {"width"=480, "height"=270, "fps"=6, "Profile"=521329048, "ppx"=237.96481, "ppy"=139.0124, "fx"=357.2274, "fy"=357.2274, "model"=4}, {"width"=480, "height"=270, "fps"=15, "Profile"=521323672, "ppx"=237.96481, "ppy"=139.0124, "fx"=357.2274, "fy"=357.2274, "model"=4}, {"width"=480, "height"=270, "fps"=30, "Profile"=521332632, "ppx"=237.96481, "ppy"=139.0124, "fx"=357.2274, "fy"=357.2274, "model"=4}, {"width"=480, "height"=270, "fps"=60, "Profile"=521337496, "ppx"=237.96481, "ppy"=139.0124, "fx"=357.2274, "fy"=357.2274, "model"=4}, {"width"=480, "height"=270, "fps"=90, "Profile"=521326232, "ppx"=237.96481, "ppy"=139.0124, "fx"=357.2274, "fy"=357.2274, "model"=4}, {"width"=640, "height"=360, "fps"=6, "Profile"=521353112, "ppx"=317.2864, "ppy"=185.34987, "fx"=476.3032, "fy"=476.3032, "model"=4}, {"width"=640, "height"=360, "fps"=15, "Profile"=521347992, "ppx"=317.2864, "ppy"=185.34987, "fx"=476.3032, "fy"=476.3032, "model"=4}, {"width"=640, "height"=360, "fps"=30, "Profile"=521345432, "ppx"=317.2864, "ppy"=185.34987, "fx"=476.3032, "fy"=476.3032, "model"=4}, {"width"=640, "height"=360, "fps"=60, "Profile"=521332888, "ppx"=317.2864, "ppy"=185.34987, "fx"=476.3032, "fy"=476.3032, "model"=4}, {"width"=640, "height"=360, "fps"=90, "Profile"=521326744, "ppx"=317.2864, "ppy"=185.34987, "fx"=476.3032, "fy"=476.3032, "model"=4}, {"width"=640, "height"=480, "fps"=6, "Profile"=521349272, "ppx"=316.38187, "ppy"=247.13316, "fx"=635.0709, "fy"=635.0709, "model"=4}, {"width"=640, "height"=480, "fps"=15, "Profile"=521350808, "ppx"=316.38187, "ppy"=247.13316, "fx"=635.0709, "fy"=635.0709, "model"=4}, {"width"=640, "height"=480, "fps"=30, "Profile"=521350296, "ppx"=316.38187, "ppy"=247.13316, "fx"=635.0709, "fy"=635.0709, "model"=4}, {"width"=640, "height"=480, "fps"=60, "Profile"=521345944, "ppx"=316.38187, "ppy"=247.13316, "fx"=635.0709, "fy"=635.0709, "model"=4}, {"width"=640, "height"=480, "fps"=90, "Profile"=521351576, "ppx"=316.38187, "ppy"=247.13316, "fx"=635.0709, "fy"=635.0709, "model"=4}, {"width"=848, "height"=480, "fps"=6, "Profile"=521610680, "ppx"=420.38187, "ppy"=247.13316, "fx"=635.0709, "fy"=635.0709, "model"=4}, {"width"=848, "height"=480, "fps"=15, "Profile"=521617592, "ppx"=420.38187, "ppy"=247.13316, "fx"=635.0709, "fy"=635.0709, "model"=4}, {"width"=848, "height"=480, "fps"=30, "Profile"=521343640, "ppx"=420.38187, "ppy"=247.13316, "fx"=635.0709, "fy"=635.0709, "model"=4}, {"width"=848, "height"=480, "fps"=60, "Profile"=521354136, "ppx"=420.38187, "ppy"=247.13316, "fx"=635.0709, "fy"=635.0709, "model"=4}, {"width"=848, "height"=480, "fps"=90, "Profile"=521351064, "ppx"=420.38187, "ppy"=247.13316, "fx"=635.0709, "fy"=635.0709, "model"=4}, {"width"=1280, "height"=720, "fps"=6, "Profile"=521617336, "ppx"=634.5728, "ppy"=370.69974, "fx"=952.6064, "fy"=952.6064, "model"=4}, {"width"=1280, "height"=720, "fps"=15, "Profile"=521604536, "ppx"=634.5728, "ppy"=370.69974, "fx"=952.6064, "fy"=952.6064, "model"=4}, {"width"=1280, "height"=720, "fps"=30, "Profile"=521605560, "ppx"=634.5728, "ppy"=370.69974, "fx"=952.6064, "fy"=952.6064, "model"=4}], 11 "Unrectified L IR":string[](array[string])=["424 x 240 @6fps", "424 x 240 @15fps", "424 x 240 @30fps", "424 x 240 @60fps", "424 x 240 @90fps", "480 x 270 @6fps", "480 x 270 @15fps", "480 x 270 @30fps", "480 x 270 @60fps", "480 x 270 @90fps", "640 x 360 @6fps", "640 x 360 @15fps", "640 x 360 @30fps", "640 x 360 @60fps", "640 x 360 @90fps", "640 x 480 @6fps", "640 x 480 @15fps", "640 x 480 @30fps", "640 x 480 @60fps", "640 x 480 @90fps", "848 x 480 @6fps", "848 x 480 @15fps", "848 x 480 @30fps", "848 x 480 @60fps", "848 x 480 @90fps", "1280 x 720 @6fps", "1280 x 720 @15fps", "1280 x 720 @30fps"], 12 "IR Right Array":string[](array[string])=["424 x 240 @6fps", "424 x 240 @15fps", "424 x 240 @30fps", "424 x 240 @60fps", "424 x 240 @90fps", "480 x 270 @6fps", "480 x 270 @15fps", "480 x 270 @30fps", "480 x 270 @60fps", "480 x 270 @90fps", "640 x 360 @6fps", "640 x 360 @15fps", "640 x 360 @30fps", "640 x 360 @60fps", "640 x 360 @90fps", "640 x 480 @6fps", "640 x 480 @15fps", "640 x 480 @30fps", "640 x 480 @60fps", "640 x 480 @90fps", "848 x 480 @6fps", "848 x 480 @15fps", "848 x 480 @30fps", "848 x 480 @60fps", "848 x 480 @90fps", "1280 x 720 @6fps", "1280 x 720 @15fps", "1280 x 720 @30fps", "1920 x 1080 @15fps", "1920 x 1080 @25fps"], 13 "Unrectified R  IR":T1(array[cluster])=[{"width"=424, "height"=240, "fps"=6, "Profile"=521292696, "ppx"=210.19093, "ppy"=123.56658, "fx"=317.53546, "fy"=317.53546, "model"=4}, {"width"=424, "height"=240, "fps"=15, "Profile"=521302424, "ppx"=210.19093, "ppy"=123.56658, "fx"=317.53546, "fy"=317.53546, "model"=4}, {"width"=424, "height"=240, "fps"=30, "Profile"=521300120, "ppx"=210.19093, "ppy"=123.56658, "fx"=317.53546, "fy"=317.53546, "model"=4}, {"width"=424, "height"=240, "fps"=60, "Profile"=521291928, "ppx"=210.19093, "ppy"=123.56658, "fx"=317.53546, "fy"=317.53546, "model"=4}, {"width"=424, "height"=240, "fps"=90, "Profile"=521301912, "ppx"=210.19093, "ppy"=123.56658, "fx"=317.53546, "fy"=317.53546, "model"=4}, {"width"=480, "height"=270, "fps"=6, "Profile"=521303704, "ppx"=237.96481, "ppy"=139.0124, "fx"=357.2274, "fy"=357.2274, "model"=4}, {"width"=480, "height"=270, "fps"=15, "Profile"=521304984, "ppx"=237.96481, "ppy"=139.0124, "fx"=357.2274, "fy"=357.2274, "model"=4}, {"width"=480, "height"=270, "fps"=30, "Profile"=521301144, "ppx"=237.96481, "ppy"=139.0124, "fx"=357.2274, "fy"=357.2274, "model"=4}, {"width"=480, "height"=270, "fps"=60, "Profile"=521300376, "ppx"=237.96481, "ppy"=139.0124, "fx"=357.2274, "fy"=357.2274, "model"=4}, {"width"=480, "height"=270, "fps"=90, "Profile"=521297560, "ppx"=237.96481, "ppy"=139.0124, "fx"=357.2274, "fy"=357.2274, "model"=4}, {"width"=640, "height"=360, "fps"=6, "Profile"=521313944, "ppx"=317.2864, "ppy"=185.34987, "fx"=476.3032, "fy"=476.3032, "model"=4}, {"width"=640, "height"=360, "fps"=15, "Profile"=521308312, "ppx"=317.2864, "ppy"=185.34987, "fx"=476.3032, "fy"=476.3032, "model"=4}, {"width"=640, "height"=360, "fps"=30, "Profile"=521293720, "ppx"=317.2864, "ppy"=185.34987, "fx"=476.3032, "fy"=476.3032, "model"=4}, {"width"=640, "height"=360, "fps"=60, "Profile"=521292952, "ppx"=317.2864, "ppy"=185.34987, "fx"=476.3032, "fy"=476.3032, "model"=4}, {"width"=640, "height"=360, "fps"=90, "Profile"=521306520, "ppx"=317.2864, "ppy"=185.34987, "fx"=476.3032, "fy"=476.3032, "model"=4}, {"width"=640, "height"=480, "fps"=6, "Profile"=521307800, "ppx"=316.38187, "ppy"=247.13316, "fx"=635.0709, "fy"=635.0709, "model"=4}, {"width"=640, "height"=480, "fps"=15, "Profile"=521316760, "ppx"=316.38187, "ppy"=247.13316, "fx"=635.0709, "fy"=635.0709, "model"=4}, {"width"=640, "height"=480, "fps"=30, "Profile"=521309848, "ppx"=316.38187, "ppy"=247.13316, "fx"=635.0709, "fy"=635.0709, "model"=4}, {"width"=640, "height"=480, "fps"=60, "Profile"=521318552, "ppx"=316.38187, "ppy"=247.13316, "fx"=635.0709, "fy"=635.0709, "model"=4}, {"width"=640, "height"=480, "fps"=90, "Profile"=521313432, "ppx"=316.38187, "ppy"=247.13316, "fx"=635.0709, "fy"=635.0709, "model"=4}, {"width"=848, "height"=480, "fps"=6, "Profile"=521308824, "ppx"=420.38187, "ppy"=247.13316, "fx"=635.0709, "fy"=635.0709, "model"=4}, {"width"=848, "height"=480, "fps"=15, "Profile"=521308056, "ppx"=420.38187, "ppy"=247.13316, "fx"=635.0709, "fy"=635.0709, "model"=4}, {"width"=848, "height"=480, "fps"=30, "Profile"=521320856, "ppx"=420.38187, "ppy"=247.13316, "fx"=635.0709, "fy"=635.0709, "model"=4}, {"width"=848, "height"=480, "fps"=60, "Profile"=521318040, "ppx"=420.38187, "ppy"=247.13316, "fx"=635.0709, "fy"=635.0709, "model"=4}, {"width"=848, "height"=480, "fps"=90, "Profile"=521322392, "ppx"=420.38187, "ppy"=247.13316, "fx"=635.0709, "fy"=635.0709, "model"=4}, {"width"=1280, "height"=720, "fps"=6, "Profile"=521315224, "ppx"=634.5728, "ppy"=370.69974, "fx"=952.6064, "fy"=952.6064, "model"=4}, {"width"=1280, "height"=720, "fps"=15, "Profile"=521316248, "ppx"=634.5728, "ppy"=370.69974, "fx"=952.6064, "fy"=952.6064, "model"=4}, {"width"=1280, "height"=720, "fps"=30, "Profile"=521319832, "ppx"=634.5728, "ppy"=370.69974, "fx"=952.6064, "fy"=952.6064, "model"=4}], 14 "IR Right":T1(array[cluster])=[{"width"=424, "height"=240, "fps"=6, "Profile"=521602232, "ppx"=210.19093, "ppy"=123.56658, "fx"=317.53546, "fy"=317.53546, "model"=4}, {"width"=424, "height"=240, "fps"=15, "Profile"=521611192, "ppx"=210.19093, "ppy"=123.56658, "fx"=317.53546, "fy"=317.53546, "model"=4}, {"width"=424, "height"=240, "fps"=30, "Profile"=521614264, "ppx"=210.19093, "ppy"=123.56658, "fx"=317.53546, "fy"=317.53546, "model"=4}, {"width"=424, "height"=240, "fps"=60, "Profile"=521614008, "ppx"=210.19093, "ppy"=123.56658, "fx"=317.53546, "fy"=317.53546, "model"=4}, {"width"=424, "height"=240, "fps"=90, "Profile"=521601976, "ppx"=210.19093, "ppy"=123.56658, "fx"=317.53546, "fy"=317.53546, "model"=4}, {"width"=480, "height"=270, "fps"=6, "Profile"=521602488, "ppx"=237.96481, "ppy"=139.0124, "fx"=357.2274, "fy"=357.2274, "model"=4}, {"width"=480, "height"=270, "fps"=15, "Profile"=521610936, "ppx"=237.96481, "ppy"=139.0124, "fx"=357.2274, "fy"=357.2274, "model"=4}, {"width"=480, "height"=270, "fps"=30, "Profile"=521605048, "ppx"=237.96481, "ppy"=139.0124, "fx"=357.2274, "fy"=357.2274, "model"=4}, {"width"=480, "height"=270, "fps"=60, "Profile"=521603000, "ppx"=237.96481, "ppy"=139.0124, "fx"=357.2274, "fy"=357.2274, "model"=4}, {"width"=480, "height"=270, "fps"=90, "Profile"=521612216, "ppx"=237.96481, "ppy"=139.0124, "fx"=357.2274, "fy"=357.2274, "model"=4}, {"width"=640, "height"=360, "fps"=6, "Profile"=521611448, "ppx"=317.2864, "ppy"=185.34987, "fx"=476.3032, "fy"=476.3032, "model"=4}, {"width"=640, "height"=360, "fps"=15, "Profile"=521613496, "ppx"=317.2864, "ppy"=185.34987, "fx"=476.3032, "fy"=476.3032, "model"=4}, {"width"=640, "height"=360, "fps"=30, "Profile"=521604792, "ppx"=317.2864, "ppy"=185.34987, "fx"=476.3032, "fy"=476.3032, "model"=4}, {"width"=640, "height"=360, "fps"=60, "Profile"=521606072, "ppx"=317.2864, "ppy"=185.34987, "fx"=476.3032, "fy"=476.3032, "model"=4}, {"width"=640, "height"=360, "fps"=90, "Profile"=521609656, "ppx"=317.2864, "ppy"=185.34987, "fx"=476.3032, "fy"=476.3032, "model"=4}, {"width"=640, "height"=480, "fps"=6, "Profile"=521608376, "ppx"=316.38187, "ppy"=247.13316, "fx"=635.0709, "fy"=635.0709, "model"=4}, {"width"=640, "height"=480, "fps"=15, "Profile"=521608120, "ppx"=316.38187, "ppy"=247.13316, "fx"=635.0709, "fy"=635.0709, "model"=4}, {"width"=640, "height"=480, "fps"=30, "Profile"=521607352, "ppx"=316.38187, "ppy"=247.13316, "fx"=635.0709, "fy"=635.0709, "model"=4}, {"width"=640, "height"=480, "fps"=60, "Profile"=521615032, "ppx"=316.38187, "ppy"=247.13316, "fx"=635.0709, "fy"=635.0709, "model"=4}, {"width"=640, "height"=480, "fps"=90, "Profile"=521605304, "ppx"=316.38187, "ppy"=247.13316, "fx"=635.0709, "fy"=635.0709, "model"=4}, {"width"=848, "height"=480, "fps"=6, "Profile"=521616568, "ppx"=420.38187, "ppy"=247.13316, "fx"=635.0709, "fy"=635.0709, "model"=4}, {"width"=848, "height"=480, "fps"=15, "Profile"=521615288, "ppx"=420.38187, "ppy"=247.13316, "fx"=635.0709, "fy"=635.0709, "model"=4}, {"width"=848, "height"=480, "fps"=30, "Profile"=521609144, "ppx"=420.38187, "ppy"=247.13316, "fx"=635.0709, "fy"=635.0709, "model"=4}, {"width"=848, "height"=480, "fps"=60, "Profile"=521611960, "ppx"=420.38187, "ppy"=247.13316, "fx"=635.0709, "fy"=635.0709, "model"=4}, {"width"=848, "height"=480, "fps"=90, "Profile"=521614776, "ppx"=420.38187, "ppy"=247.13316, "fx"=635.0709, "fy"=635.0709, "model"=4}, {"width"=1280, "height"=720, "fps"=6, "Profile"=521608888, "ppx"=634.5728, "ppy"=370.69974, "fx"=952.6064, "fy"=952.6064, "model"=4}, {"width"=1280, "height"=720, "fps"=15, "Profile"=521616824, "ppx"=634.5728, "ppy"=370.69974, "fx"=952.6064, "fy"=952.6064, "model"=4}, {"width"=1280, "height"=720, "fps"=30, "Profile"=521615544, "ppx"=634.5728, "ppy"=370.69974, "fx"=952.6064, "fy"=952.6064, "model"=4}, {"width"=1920, "height"=1080, "fps"=15, "Profile"=521628088, "ppx"=951.85925, "ppy"=556.0496, "fx"=1428.9095, "fy"=1428.9095, "model"=4}, {"width"=1920, "height"=1080, "fps"=25, "Profile"=521608632, "ppx"=951.85925, "ppy"=556.0496, "fx"=1428.9095, "fy"=1428.9095, "model"=4}], 15 "Color Left Array":string[](array[string])=["424 x 240 @6fps", "424 x 240 @15fps", "424 x 240 @30fps", "424 x 240 @60fps", "424 x 240 @90fps", "480 x 270 @6fps", "480 x 270 @15fps", "480 x 270 @30fps", "480 x 270 @60fps", "480 x 270 @90fps", "640 x 360 @6fps", "640 x 360 @15fps", "640 x 360 @30fps", "640 x 360 @60fps", "640 x 360 @90fps", "640 x 480 @6fps", "640 x 480 @15fps", "640 x 480 @30fps", "640 x 480 @60fps", "640 x 480 @90fps", "848 x 480 @6fps", "848 x 480 @15fps", "848 x 480 @30fps", "848 x 480 @60fps", "848 x 480 @90fps", "1280 x 720 @6fps", "1280 x 720 @15fps", "1280 x 720 @30fps"])   [LabVIEW 2017, in "libRealSense3.lvlib"]
doc: "This helper VI is used to decode the numerous streams, and parse them into arrays of Depth, Color Left, IR left, IR Right, Unrectified L, Unrectified R."
uses:
  <vilib>/addons/RealSense/libRealSense3.lvlib
panel:
  # "RS3 Decode Depth Streams"
  # "(C) Intel Corp.,  AGJ 2017"
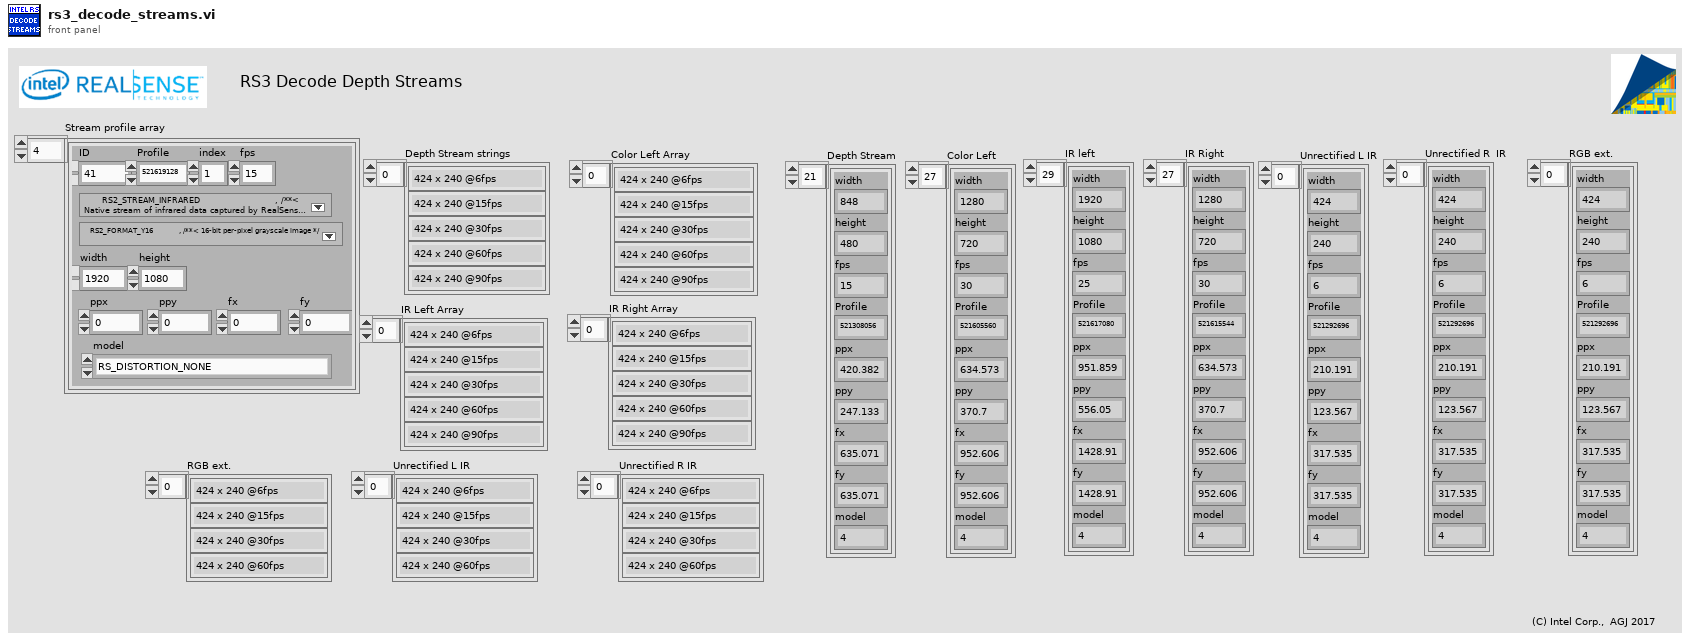
[diagram p1: front panel]
types:
  T1 = cluster{"width":i32, "height":i32, "fps":i32, "Profile":u64, "ppx":sgl, "ppy":sgl, "fx":sgl, "fy":sgl, "model":u32}[]
  T2 = cluster{"ID":i32, "Profile":u64, "fps":i32, "RS Stream":u16, "RS Format":u16, "index":u16, "width":i32, "height":i32, "ppx":sgl, "ppy":sgl, "fx":sgl, "fy":sgl, "model":u32}[]
  T3 = cluster{"width":i32, "height":i32, "fps":i32, "Profile":u64, "ppx":sgl, "ppy":sgl, "fx":sgl, "fy":sgl, "model":u32}
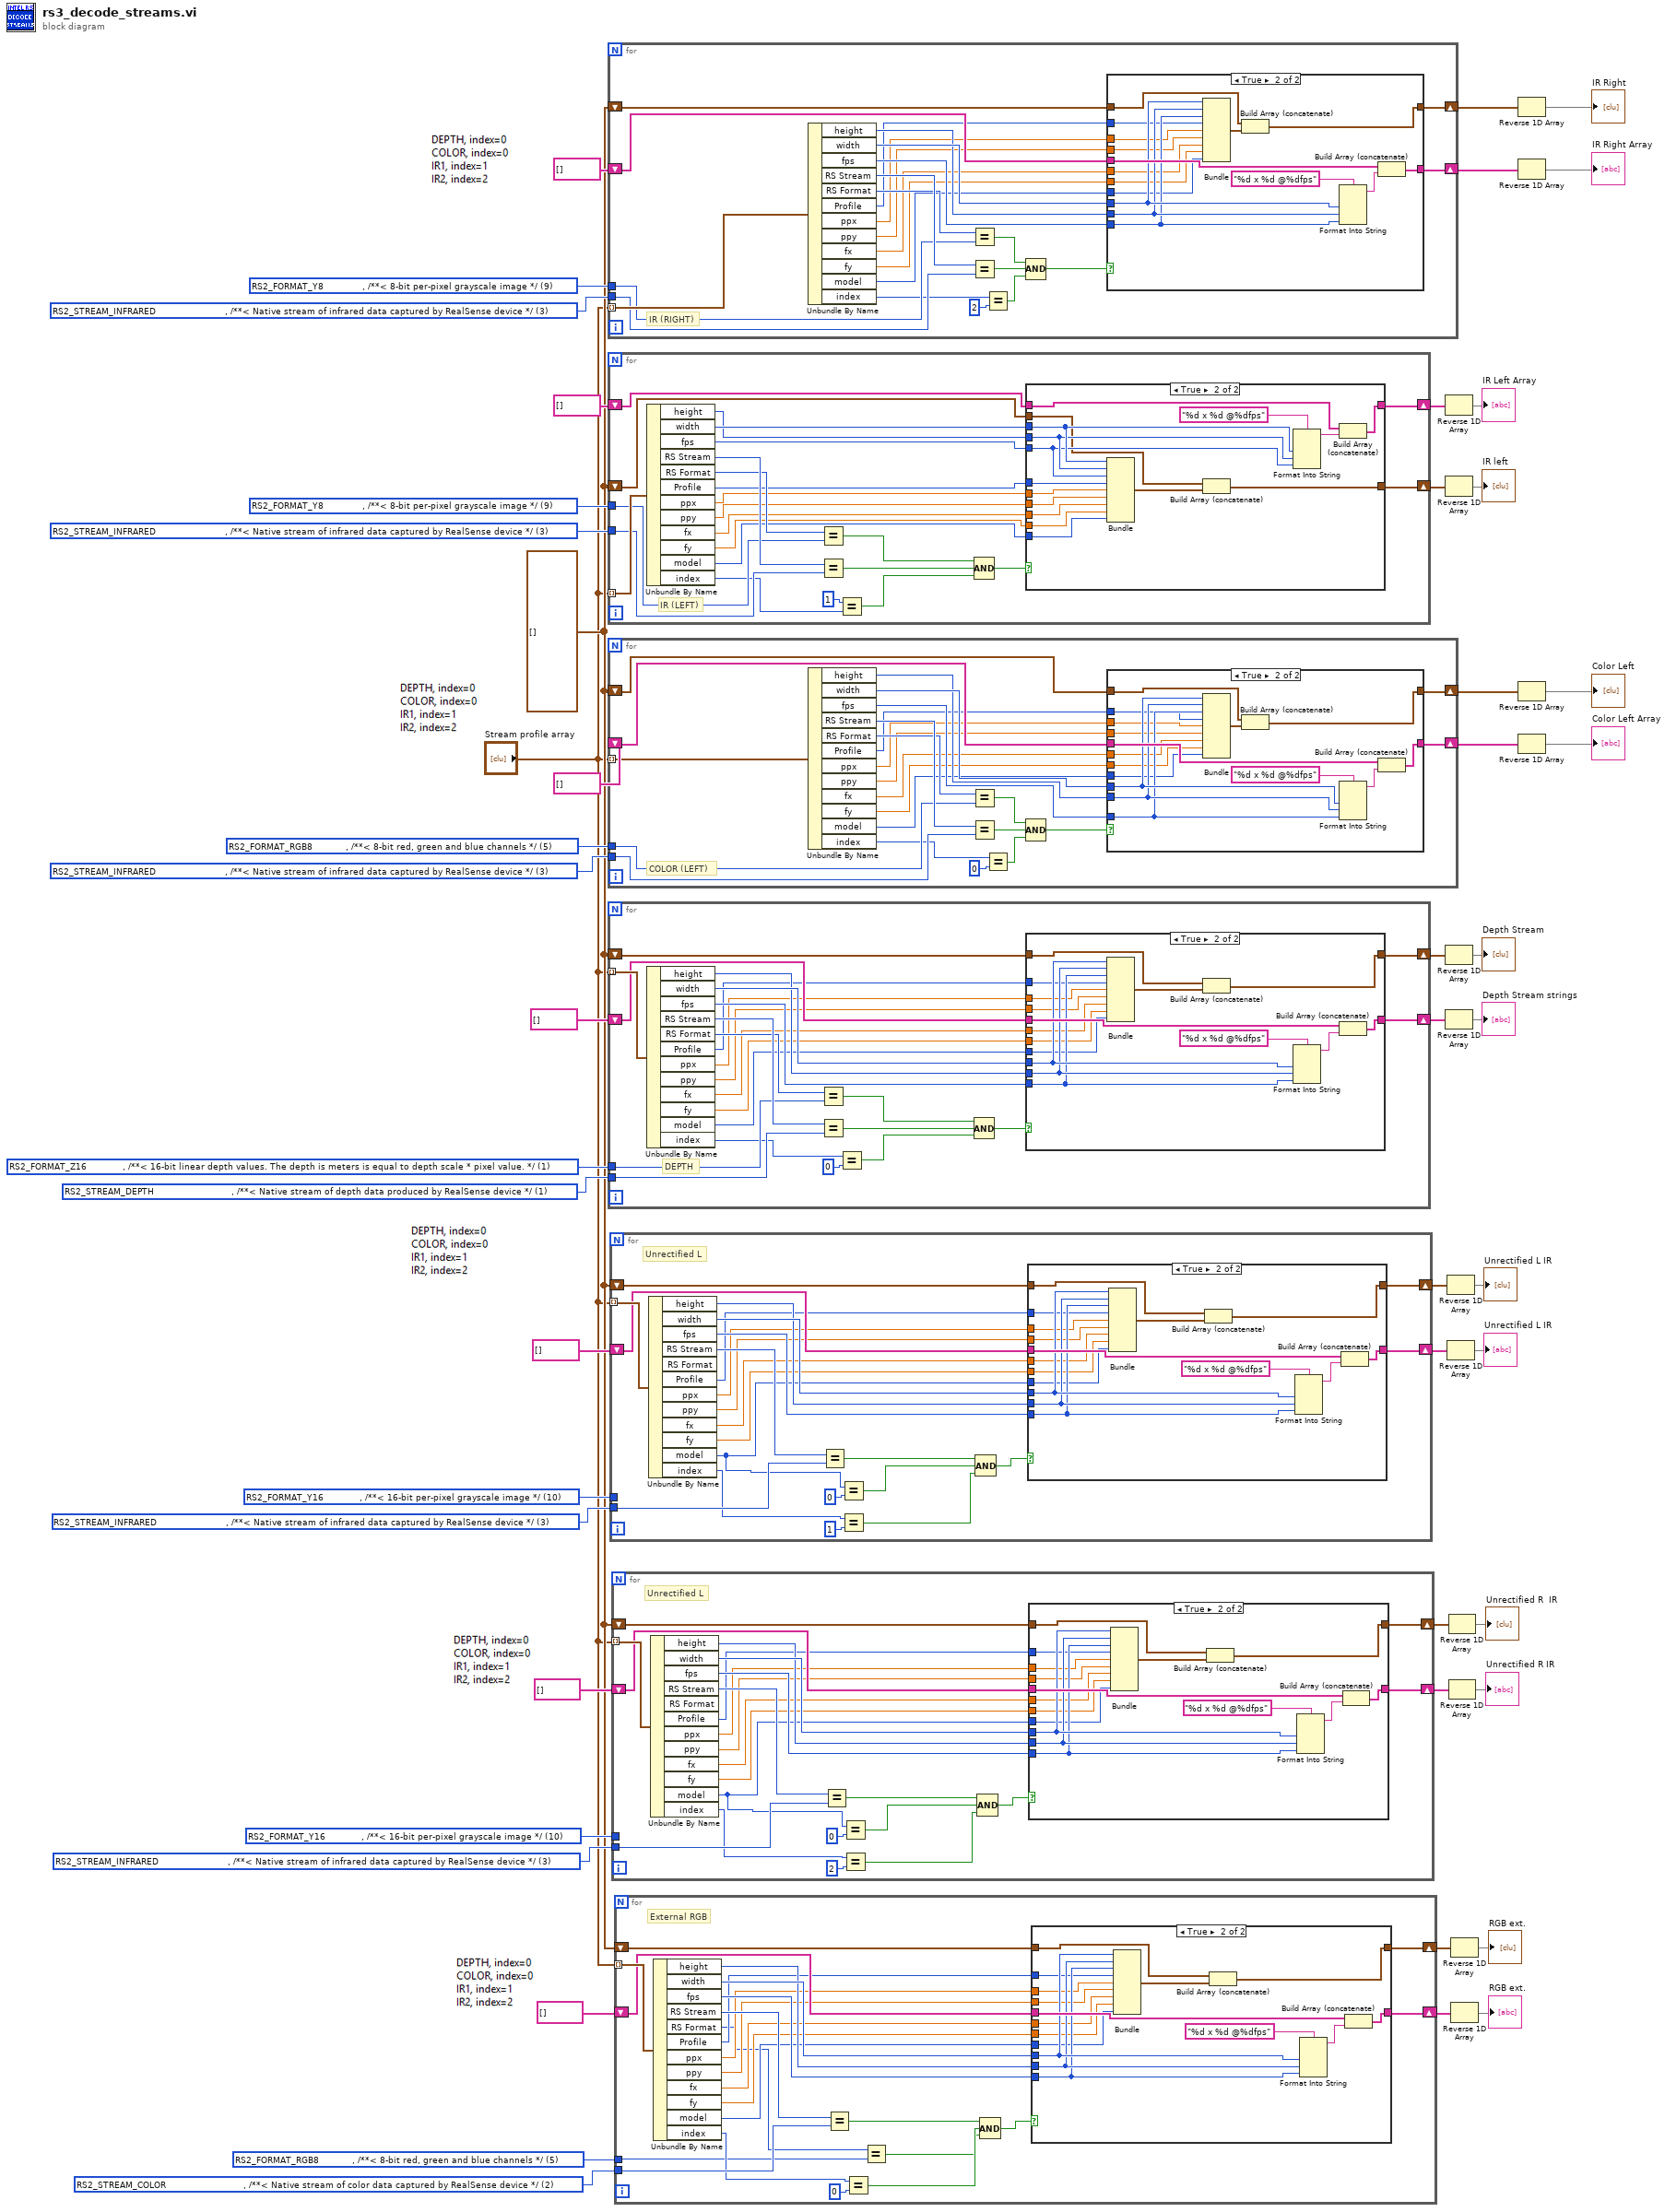
[diagram p0: block diagram]
diagram:
  w5 = u16 5 items=["    RS2_FORMAT_ANY             , /**< When passed to enable stream, librealsense will try to provide best suited format */", "    RS2_FORMAT_Z16             , /**< 16-bit linear depth values. The depth is meters is equal to depth scale * pixel value. */", "    RS2_FORMAT_DISPARITY16     , /**< 16-bit linear disparity values. The depth in meters is equal to depth scale / pixel value. */", "    RS2_FORMAT_XYZ32F          , /**< 32-bit floating point 3D coordinates. */", "    RS2_FORMAT_YUYV            , /**< Standard YUV pixel format as described in https://en.wikipedia.org/wiki/YUV */", "    RS2_FORMAT_RGB8            , /**< 8-bit red, green and blue channels */", "    RS2_FORMAT_BGR8            , /**< 8-bit blue, green, and red channels -- suitable for OpenCV */", "    RS2_FORMAT_RGBA8           , /**< 8-bit red, green and blue channels + constant alpha channel equal to FF */", "    RS2_FORMAT_BGRA8           , /**< 8-bit blue, green, and red channels + constant alpha channel equal to FF */", "    RS2_FORMAT_Y8              , /**< 8-bit per-pixel grayscale image */", "    RS2_FORMAT_Y16             , /**< 16-bit per-pixel grayscale image */", "    RS2_FORMAT_RAW10           , /**< Four 10-bit luminance values encoded into a 5-byte macropixel */", "    RS2_FORMAT_RAW16           , /**< 16-bit raw image */", "    RS2_FORMAT_RAW8            , /**< 8-bit raw image */", "    RS2_FORMAT_UYVY            , /**< Similar to the standard YUYV pixel format, but packed in a different order */", "    RS2_FORMAT_MOTION_RAW      , /**< Raw data from the motion sensor */", "    RS2_FORMAT_MOTION_XYZ32F   , /**< Motion data packed as 3 32-bit float values, for X, Y, and Z axis */", "    RS2_FORMAT_GPIO_RAW        , /**< Raw data from the external sensors hooked to one of the GPIO's */", "    RS2_FORMAT_COUNT             /**< Number of enumeration values. Not a valid input: intended to be used in for-loops. */"] ("RS Format")
  w4 = u16 2 items=["    RS2_STREAM_ANY,", "    RS2_STREAM_DEPTH                            , /**< Native stream of depth data produced by RealSense device */", "    RS2_STREAM_COLOR                            , /**< Native stream of color data captured by RealSense device */", "    RS2_STREAM_INFRARED                         , /**< Native stream of infrared data captured by RealSense device */", "    RS2_STREAM_FISHEYE                          , /**< Native stream of fish-eye (wide) data captured from the dedicate motion camera */", "    RS2_STREAM_GYRO                             , /**< Native stream of gyroscope motion data produced by RealSense device */", "    RS2_STREAM_ACCEL                            , /**< Native stream of accelerometer motion data produced by RealSense device */", "    RS2_STREAM_GPIO                             , /**< Signals from external device connected through GPIO */", "    RS2_STREAM_COUNT"] ("RS Stream")
  w17 = u16 10 items=["    RS2_FORMAT_ANY             , /**< When passed to enable stream, librealsense will try to provide best suited format */", "    RS2_FORMAT_Z16             , /**< 16-bit linear depth values. The depth is meters is equal to depth scale * pixel value. */", "    RS2_FORMAT_DISPARITY16     , /**< 16-bit linear disparity values. The depth in meters is equal to depth scale / pixel value. */", "    RS2_FORMAT_XYZ32F          , /**< 32-bit floating point 3D coordinates. */", "    RS2_FORMAT_YUYV            , /**< Standard YUV pixel format as described in https://en.wikipedia.org/wiki/YUV */", "    RS2_FORMAT_RGB8            , /**< 8-bit red, green and blue channels */", "    RS2_FORMAT_BGR8            , /**< 8-bit blue, green, and red channels -- suitable for OpenCV */", "    RS2_FORMAT_RGBA8           , /**< 8-bit red, green and blue channels + constant alpha channel equal to FF */", "    RS2_FORMAT_BGRA8           , /**< 8-bit blue, green, and red channels + constant alpha channel equal to FF */", "    RS2_FORMAT_Y8              , /**< 8-bit per-pixel grayscale image */", "    RS2_FORMAT_Y16             , /**< 16-bit per-pixel grayscale image */", "    RS2_FORMAT_RAW10           , /**< Four 10-bit luminance values encoded into a 5-byte macropixel */", "    RS2_FORMAT_RAW16           , /**< 16-bit raw image */", "    RS2_FORMAT_RAW8            , /**< 8-bit raw image */", "    RS2_FORMAT_UYVY            , /**< Similar to the standard YUYV pixel format, but packed in a different order */", "    RS2_FORMAT_MOTION_RAW      , /**< Raw data from the motion sensor */", "    RS2_FORMAT_MOTION_XYZ32F   , /**< Motion data packed as 3 32-bit float values, for X, Y, and Z axis */", "    RS2_FORMAT_GPIO_RAW        , /**< Raw data from the external sensors hooked to one of the GPIO's */", "    RS2_FORMAT_COUNT             /**< Number of enumeration values. Not a valid input: intended to be used in for-loops. */"] ("RS Format")
  w18 = u16 3 items=["    RS2_STREAM_ANY,", "    RS2_STREAM_DEPTH                            , /**< Native stream of depth data produced by RealSense device */", "    RS2_STREAM_COLOR                            , /**< Native stream of color data captured by RealSense device */", "    RS2_STREAM_INFRARED                         , /**< Native stream of infrared data captured by RealSense device */", "    RS2_STREAM_FISHEYE                          , /**< Native stream of fish-eye (wide) data captured from the dedicate motion camera */", "    RS2_STREAM_GYRO                             , /**< Native stream of gyroscope motion data produced by RealSense device */", "    RS2_STREAM_ACCEL                            , /**< Native stream of accelerometer motion data produced by RealSense device */", "    RS2_STREAM_GPIO                             , /**< Signals from external device connected through GPIO */", "    RS2_STREAM_COUNT"] ("RS Stream")
  w22 = u16 10 items=["    RS2_FORMAT_ANY             , /**< When passed to enable stream, librealsense will try to provide best suited format */", "    RS2_FORMAT_Z16             , /**< 16-bit linear depth values. The depth is meters is equal to depth scale * pixel value. */", "    RS2_FORMAT_DISPARITY16     , /**< 16-bit linear disparity values. The depth in meters is equal to depth scale / pixel value. */", "    RS2_FORMAT_XYZ32F          , /**< 32-bit floating point 3D coordinates. */", "    RS2_FORMAT_YUYV            , /**< Standard YUV pixel format as described in https://en.wikipedia.org/wiki/YUV */", "    RS2_FORMAT_RGB8            , /**< 8-bit red, green and blue channels */", "    RS2_FORMAT_BGR8            , /**< 8-bit blue, green, and red channels -- suitable for OpenCV */", "    RS2_FORMAT_RGBA8           , /**< 8-bit red, green and blue channels + constant alpha channel equal to FF */", "    RS2_FORMAT_BGRA8           , /**< 8-bit blue, green, and red channels + constant alpha channel equal to FF */", "    RS2_FORMAT_Y8              , /**< 8-bit per-pixel grayscale image */", "    RS2_FORMAT_Y16             , /**< 16-bit per-pixel grayscale image */", "    RS2_FORMAT_RAW10           , /**< Four 10-bit luminance values encoded into a 5-byte macropixel */", "    RS2_FORMAT_RAW16           , /**< 16-bit raw image */", "    RS2_FORMAT_RAW8            , /**< 8-bit raw image */", "    RS2_FORMAT_UYVY            , /**< Similar to the standard YUYV pixel format, but packed in a different order */", "    RS2_FORMAT_MOTION_RAW      , /**< Raw data from the motion sensor */", "    RS2_FORMAT_MOTION_XYZ32F   , /**< Motion data packed as 3 32-bit float values, for X, Y, and Z axis */", "    RS2_FORMAT_GPIO_RAW        , /**< Raw data from the external sensors hooked to one of the GPIO's */", "    RS2_FORMAT_COUNT             /**< Number of enumeration values. Not a valid input: intended to be used in for-loops. */"] ("RS Format")
  w21 = u16 3 items=["    RS2_STREAM_ANY,", "    RS2_STREAM_DEPTH                            , /**< Native stream of depth data produced by RealSense device */", "    RS2_STREAM_COLOR                            , /**< Native stream of color data captured by RealSense device */", "    RS2_STREAM_INFRARED                         , /**< Native stream of infrared data captured by RealSense device */", "    RS2_STREAM_FISHEYE                          , /**< Native stream of fish-eye (wide) data captured from the dedicate motion camera */", "    RS2_STREAM_GYRO                             , /**< Native stream of gyroscope motion data produced by RealSense device */", "    RS2_STREAM_ACCEL                            , /**< Native stream of accelerometer motion data produced by RealSense device */", "    RS2_STREAM_GPIO                             , /**< Signals from external device connected through GPIO */", "    RS2_STREAM_COUNT"] ("RS Stream")
  w32 = u16 3 items=["    RS2_STREAM_ANY,", "    RS2_STREAM_DEPTH                            , /**< Native stream of depth data produced by RealSense device */", "    RS2_STREAM_COLOR                            , /**< Native stream of color data captured by RealSense device */", "    RS2_STREAM_INFRARED                         , /**< Native stream of infrared data captured by RealSense device */", "    RS2_STREAM_FISHEYE                          , /**< Native stream of fish-eye (wide) data captured from the dedicate motion camera */", "    RS2_STREAM_GYRO                             , /**< Native stream of gyroscope motion data produced by RealSense device */", "    RS2_STREAM_ACCEL                            , /**< Native stream of accelerometer motion data produced by RealSense device */", "    RS2_STREAM_GPIO                             , /**< Signals from external device connected through GPIO */", "    RS2_STREAM_COUNT"] ("RS Stream")
  w31 = u16 9 items=["    RS2_FORMAT_ANY             , /**< When passed to enable stream, librealsense will try to provide best suited format */", "    RS2_FORMAT_Z16             , /**< 16-bit linear depth values. The depth is meters is equal to depth scale * pixel value. */", "    RS2_FORMAT_DISPARITY16     , /**< 16-bit linear disparity values. The depth in meters is equal to depth scale / pixel value. */", "    RS2_FORMAT_XYZ32F          , /**< 32-bit floating point 3D coordinates. */", "    RS2_FORMAT_YUYV            , /**< Standard YUV pixel format as described in https://en.wikipedia.org/wiki/YUV */", "    RS2_FORMAT_RGB8            , /**< 8-bit red, green and blue channels */", "    RS2_FORMAT_BGR8            , /**< 8-bit blue, green, and red channels -- suitable for OpenCV */", "    RS2_FORMAT_RGBA8           , /**< 8-bit red, green and blue channels + constant alpha channel equal to FF */", "    RS2_FORMAT_BGRA8           , /**< 8-bit blue, green, and red channels + constant alpha channel equal to FF */", "    RS2_FORMAT_Y8              , /**< 8-bit per-pixel grayscale image */", "    RS2_FORMAT_Y16             , /**< 16-bit per-pixel grayscale image */", "    RS2_FORMAT_RAW10           , /**< Four 10-bit luminance values encoded into a 5-byte macropixel */", "    RS2_FORMAT_RAW16           , /**< 16-bit raw image */", "    RS2_FORMAT_RAW8            , /**< 8-bit raw image */", "    RS2_FORMAT_UYVY            , /**< Similar to the standard YUYV pixel format, but packed in a different order */", "    RS2_FORMAT_MOTION_RAW      , /**< Raw data from the motion sensor */", "    RS2_FORMAT_MOTION_XYZ32F   , /**< Motion data packed as 3 32-bit float values, for X, Y, and Z axis */", "    RS2_FORMAT_GPIO_RAW        , /**< Raw data from the external sensors hooked to one of the GPIO's */", "    RS2_FORMAT_COUNT             /**< Number of enumeration values. Not a valid input: intended to be used in for-loops. */"] ("RS Format")
  w33 = u16 3 items=["    RS2_STREAM_ANY,", "    RS2_STREAM_DEPTH                            , /**< Native stream of depth data produced by RealSense device */", "    RS2_STREAM_COLOR                            , /**< Native stream of color data captured by RealSense device */", "    RS2_STREAM_INFRARED                         , /**< Native stream of infrared data captured by RealSense device */", "    RS2_STREAM_FISHEYE                          , /**< Native stream of fish-eye (wide) data captured from the dedicate motion camera */", "    RS2_STREAM_GYRO                             , /**< Native stream of gyroscope motion data produced by RealSense device */", "    RS2_STREAM_ACCEL                            , /**< Native stream of accelerometer motion data produced by RealSense device */", "    RS2_STREAM_GPIO                             , /**< Signals from external device connected through GPIO */", "    RS2_STREAM_COUNT"] ("RS Stream")
  w34 = u16 9 items=["    RS2_FORMAT_ANY             , /**< When passed to enable stream, librealsense will try to provide best suited format */", "    RS2_FORMAT_Z16             , /**< 16-bit linear depth values. The depth is meters is equal to depth scale * pixel value. */", "    RS2_FORMAT_DISPARITY16     , /**< 16-bit linear disparity values. The depth in meters is equal to depth scale / pixel value. */", "    RS2_FORMAT_XYZ32F          , /**< 32-bit floating point 3D coordinates. */", "    RS2_FORMAT_YUYV            , /**< Standard YUV pixel format as described in https://en.wikipedia.org/wiki/YUV */", "    RS2_FORMAT_RGB8            , /**< 8-bit red, green and blue channels */", "    RS2_FORMAT_BGR8            , /**< 8-bit blue, green, and red channels -- suitable for OpenCV */", "    RS2_FORMAT_RGBA8           , /**< 8-bit red, green and blue channels + constant alpha channel equal to FF */", "    RS2_FORMAT_BGRA8           , /**< 8-bit blue, green, and red channels + constant alpha channel equal to FF */", "    RS2_FORMAT_Y8              , /**< 8-bit per-pixel grayscale image */", "    RS2_FORMAT_Y16             , /**< 16-bit per-pixel grayscale image */", "    RS2_FORMAT_RAW10           , /**< Four 10-bit luminance values encoded into a 5-byte macropixel */", "    RS2_FORMAT_RAW16           , /**< 16-bit raw image */", "    RS2_FORMAT_RAW8            , /**< 8-bit raw image */", "    RS2_FORMAT_UYVY            , /**< Similar to the standard YUYV pixel format, but packed in a different order */", "    RS2_FORMAT_MOTION_RAW      , /**< Raw data from the motion sensor */", "    RS2_FORMAT_MOTION_XYZ32F   , /**< Motion data packed as 3 32-bit float values, for X, Y, and Z axis */", "    RS2_FORMAT_GPIO_RAW        , /**< Raw data from the external sensors hooked to one of the GPIO's */", "    RS2_FORMAT_COUNT             /**< Number of enumeration values. Not a valid input: intended to be used in for-loops. */"] ("RS Format")
  w2 = T1 [] ("appended array")
  w45 = u16 3 items=["    RS2_STREAM_ANY,", "    RS2_STREAM_DEPTH                            , /**< Native stream of depth data produced by RealSense device */", "    RS2_STREAM_COLOR                            , /**< Native stream of color data captured by RealSense device */", "    RS2_STREAM_INFRARED                         , /**< Native stream of infrared data captured by RealSense device */", "    RS2_STREAM_FISHEYE                          , /**< Native stream of fish-eye (wide) data captured from the dedicate motion camera */", "    RS2_STREAM_GYRO                             , /**< Native stream of gyroscope motion data produced by RealSense device */", "    RS2_STREAM_ACCEL                            , /**< Native stream of accelerometer motion data produced by RealSense device */", "    RS2_STREAM_GPIO                             , /**< Signals from external device connected through GPIO */", "    RS2_STREAM_COUNT"] ("RS Stream")
  w44 = u16 5 items=["    RS2_FORMAT_ANY             , /**< When passed to enable stream, librealsense will try to provide best suited format */", "    RS2_FORMAT_Z16             , /**< 16-bit linear depth values. The depth is meters is equal to depth scale * pixel value. */", "    RS2_FORMAT_DISPARITY16     , /**< 16-bit linear disparity values. The depth in meters is equal to depth scale / pixel value. */", "    RS2_FORMAT_XYZ32F          , /**< 32-bit floating point 3D coordinates. */", "    RS2_FORMAT_YUYV            , /**< Standard YUV pixel format as described in https://en.wikipedia.org/wiki/YUV */", "    RS2_FORMAT_RGB8            , /**< 8-bit red, green and blue channels */", "    RS2_FORMAT_BGR8            , /**< 8-bit blue, green, and red channels -- suitable for OpenCV */", "    RS2_FORMAT_RGBA8           , /**< 8-bit red, green and blue channels + constant alpha channel equal to FF */", "    RS2_FORMAT_BGRA8           , /**< 8-bit blue, green, and red channels + constant alpha channel equal to FF */", "    RS2_FORMAT_Y8              , /**< 8-bit per-pixel grayscale image */", "    RS2_FORMAT_Y16             , /**< 16-bit per-pixel grayscale image */", "    RS2_FORMAT_RAW10           , /**< Four 10-bit luminance values encoded into a 5-byte macropixel */", "    RS2_FORMAT_RAW16           , /**< 16-bit raw image */", "    RS2_FORMAT_RAW8            , /**< 8-bit raw image */", "    RS2_FORMAT_UYVY            , /**< Similar to the standard YUYV pixel format, but packed in a different order */", "    RS2_FORMAT_MOTION_RAW      , /**< Raw data from the motion sensor */", "    RS2_FORMAT_MOTION_XYZ32F   , /**< Motion data packed as 3 32-bit float values, for X, Y, and Z axis */", "    RS2_FORMAT_GPIO_RAW        , /**< Raw data from the external sensors hooked to one of the GPIO's */", "    RS2_FORMAT_COUNT             /**< Number of enumeration values. Not a valid input: intended to be used in for-loops. */"] ("RS Format")
  w49 = u16 1 items=["    RS2_FORMAT_ANY             , /**< When passed to enable stream, librealsense will try to provide best suited format */", "    RS2_FORMAT_Z16             , /**< 16-bit linear depth values. The depth is meters is equal to depth scale * pixel value. */", "    RS2_FORMAT_DISPARITY16     , /**< 16-bit linear disparity values. The depth in meters is equal to depth scale / pixel value. */", "    RS2_FORMAT_XYZ32F          , /**< 32-bit floating point 3D coordinates. */", "    RS2_FORMAT_YUYV            , /**< Standard YUV pixel format as described in https://en.wikipedia.org/wiki/YUV */", "    RS2_FORMAT_RGB8            , /**< 8-bit red, green and blue channels */", "    RS2_FORMAT_BGR8            , /**< 8-bit blue, green, and red channels -- suitable for OpenCV */", "    RS2_FORMAT_RGBA8           , /**< 8-bit red, green and blue channels + constant alpha channel equal to FF */", "    RS2_FORMAT_BGRA8           , /**< 8-bit blue, green, and red channels + constant alpha channel equal to FF */", "    RS2_FORMAT_Y8              , /**< 8-bit per-pixel grayscale image */", "    RS2_FORMAT_Y16             , /**< 16-bit per-pixel grayscale image */", "    RS2_FORMAT_RAW10           , /**< Four 10-bit luminance values encoded into a 5-byte macropixel */", "    RS2_FORMAT_RAW16           , /**< 16-bit raw image */", "    RS2_FORMAT_RAW8            , /**< 8-bit raw image */", "    RS2_FORMAT_UYVY            , /**< Similar to the standard YUYV pixel format, but packed in a different order */", "    RS2_FORMAT_MOTION_RAW      , /**< Raw data from the motion sensor */", "    RS2_FORMAT_MOTION_XYZ32F   , /**< Motion data packed as 3 32-bit float values, for X, Y, and Z axis */", "    RS2_FORMAT_GPIO_RAW        , /**< Raw data from the external sensors hooked to one of the GPIO's */", "    RS2_FORMAT_COUNT             /**< Number of enumeration values. Not a valid input: intended to be used in for-loops. */"] ("RS Format")
  w50 = u16 1 items=["    RS2_STREAM_ANY,", "    RS2_STREAM_DEPTH                            , /**< Native stream of depth data produced by RealSense device */", "    RS2_STREAM_COLOR                            , /**< Native stream of color data captured by RealSense device */", "    RS2_STREAM_INFRARED                         , /**< Native stream of infrared data captured by RealSense device */", "    RS2_STREAM_FISHEYE                          , /**< Native stream of fish-eye (wide) data captured from the dedicate motion camera */", "    RS2_STREAM_GYRO                             , /**< Native stream of gyroscope motion data produced by RealSense device */", "    RS2_STREAM_ACCEL                            , /**< Native stream of accelerometer motion data produced by RealSense device */", "    RS2_STREAM_GPIO                             , /**< Signals from external device connected through GPIO */", "    RS2_STREAM_COUNT"] ("RS Stream")
  n1 = for {
    tunnel: "Stream profile array" -> [w75] mode=indexing
    shift-right: [w70] -> w30
    shift-left: string[] [] -> [w69]
    shift-right: [w68] -> w28
    shift-left: w2 -> [w67]
    tunnel: w32 -> [w65]
    tunnel: w31 -> [w62]
    # "IR (RIGHT)"
    n2 = Unbundle By Name(w75) -> ("height"=w72:i32, "width"=w73:i32, "fps"=w71:i32, "RS Stream"=w66:u16, "RS Format"=w63:u16, "Profile"=w60:u64, "ppx"=w59:sgl, "ppy"=w58:sgl, "fx"=w57:sgl, "fy"=w56:sgl, "model"=w55:u32, "index"=w54:u16)
    n3 = Equal?(x=w63, y=w62) -> (x = y?=w61:bool)
    n4 = Equal?(x=w66, y=w65) -> (x = y?=w64:bool)
    n5 = Equal?(x=w54, y=u16 2) -> (x = y?=w52:bool)
    n6 = Compound Arithmetic op=AND(w61, w64, w52) -> (w74:bool)
    n7 = case shown="True" w74 {
      tunnel: w73 -> [_ w89]
      tunnel: w72 -> [_ w88]
      tunnel: w71 -> [_ w87]
      tunnel: [w77 w91] -> w70
      tunnel: w69 -> [w77 w90]
      tunnel: [w76 w85] -> w68
      tunnel: w67 -> [w76 w84]
      tunnel: w60 -> [_ w83]
      tunnel: w59 -> [_ w82]
      tunnel: w58 -> [_ w81]
      tunnel: w57 -> [_ w80]
      tunnel: w56 -> [_ w79]
      tunnel: w55 -> [_ w78]
      frame False {
      }
      frame True {
        n8 = Bundle("width"=w89, "height"=w88, "fps"=w87, "Profile"=w83, "ppx"=w82, "ppy"=w81, "fx"=w80, "fy"=w79, "model"=w78) -> (w86:T3)  [unwired: 1 in]
        n9 = Build Array (concatenate)(w84, w86) -> (w85:T1)
        n10 = Format Into String(format string="%d x %d @%dfps", w89, w88, w87) -> (resulting string=w92:string)  [unwired: 2 in, 1 out]
        n11 = Build Array (concatenate)(w90, w92) -> (w91:string[])
      }
    }
  }
  n12 = for {
    tunnel: "Stream profile array" -> [w117] mode=indexing
    shift-right: [w112] -> w35
    shift-left: string[] [] -> [w111]
    shift-right: [w110] -> w37
    shift-left: w2 -> [w109]
    tunnel: w33 -> [w107]
    tunnel: w34 -> [w104]
    # "IR (LEFT)"
    n13 = Unbundle By Name(w117) -> ("height"=w114:i32, "width"=w115:i32, "fps"=w113:i32, "RS Stream"=w108:u16, "RS Format"=w105:u16, "Profile"=w103:u64, "ppx"=w102:sgl, "ppy"=w101:sgl, "fx"=w100:sgl, "fy"=w99:sgl, "model"=w98:u32, "index"=w96:u16)
    n14 = Equal?(x=w105, y=w104) -> (x = y?=w97:bool)
    n15 = Equal?(x=w108, y=w107) -> (x = y?=w106:bool)
    n16 = Equal?(x=u16 1, y=w96) -> (x = y?=w94:bool)
    n17 = Compound Arithmetic op=AND(w97, w106, w94) -> (w116:bool)
    n18 = case shown="True" w116 {
      tunnel: w115 -> [_ w131]
      tunnel: w114 -> [_ w130]
      tunnel: w113 -> [_ w129]
      tunnel: [w119 w133] -> w112
      tunnel: w111 -> [w119 w132]
      tunnel: [w118 w127] -> w110
      tunnel: w109 -> [w118 w126]
      tunnel: w103 -> [_ w125]
      tunnel: w102 -> [_ w124]
      tunnel: w101 -> [_ w123]
      tunnel: w100 -> [_ w122]
      tunnel: w99 -> [_ w121]
      tunnel: w98 -> [_ w120]
      frame False {
      }
      frame True {
        n19 = Bundle("width"=w131, "height"=w130, "fps"=w129, "Profile"=w125, "ppx"=w124, "ppy"=w123, "fx"=w122, "fy"=w121, "model"=w120) -> (w128:T3)  [unwired: 1 in]
        n20 = Build Array (concatenate)(w126, w128) -> (w127:T1)
        n21 = Format Into String(format string="%d x %d @%dfps", w131, w130, w129) -> (resulting string=w134:string)  [unwired: 2 in, 1 out]
        n22 = Build Array (concatenate)(w132, w134) -> (w133:string[])
      }
    }
  }
  n23 = for {
    tunnel: "Stream profile array" -> [w159] mode=indexing
    shift-right: [w154] -> w43
    shift-left: string[] [] -> [w153]
    shift-right: [w152] -> w41
    shift-left: w2 -> [w151]
    tunnel: w45 -> [w149]
    tunnel: w44 -> [w146]
    # "COLOR (LEFT)"
    n24 = Unbundle By Name(w159) -> ("height"=w156:i32, "width"=w157:i32, "fps"=w155:i32, "RS Stream"=w150:u16, "RS Format"=w147:u16, "Profile"=w144:u64, "ppx"=w143:sgl, "ppy"=w142:sgl, "fx"=w141:sgl, "fy"=w140:sgl, "model"=w139:u32, "index"=w138:u16)
    n25 = Equal?(x=w147, y=w146) -> (x = y?=w145:bool)
    n26 = Equal?(x=w150, y=w149) -> (x = y?=w148:bool)
    n27 = Equal?(x=w138, y=u16 0) -> (x = y?=w136:bool)
    n28 = Compound Arithmetic op=AND(w145, w148, w136) -> (w158:bool)
    n29 = case shown="True" w158 {
      tunnel: w157 -> [_ w173]
      tunnel: w156 -> [_ w172]
      tunnel: w155 -> [_ w171]
      tunnel: [w161 w175] -> w154
      tunnel: w153 -> [w161 w174]
      tunnel: [w160 w169] -> w152
      tunnel: w151 -> [w160 w168]
      tunnel: w144 -> [_ w167]
      tunnel: w143 -> [_ w166]
      tunnel: w142 -> [_ w165]
      tunnel: w141 -> [_ w164]
      tunnel: w140 -> [_ w163]
      tunnel: w139 -> [_ w162]
      frame False {
      }
      frame True {
        n30 = Bundle("width"=w173, "height"=w172, "fps"=w171, "Profile"=w167, "ppx"=w166, "ppy"=w165, "fx"=w164, "fy"=w163, "model"=w162) -> (w170:T3)  [unwired: 1 in]
        n31 = Build Array (concatenate)(w168, w170) -> (w169:T1)
        n32 = Format Into String(format string="%d x %d @%dfps", w173, w172, w171) -> (resulting string=w176:string)  [unwired: 2 in, 1 out]
        n33 = Build Array (concatenate)(w174, w176) -> (w175:string[])
      }
    }
  }
  n34 = for {
    tunnel: "Stream profile array" -> [w201] mode=indexing
    shift-right: [w196] -> w48
    shift-left: string[] [] -> [w195]
    shift-right: [w194] -> w46
    shift-left: w2 -> [w193]
    tunnel: w50 -> [w191]
    tunnel: w49 -> [w188]
    # "DEPTH"
    n35 = Unbundle By Name(w201) -> ("height"=w198:i32, "width"=w199:i32, "fps"=w197:i32, "RS Stream"=w192:u16, "RS Format"=w189:u16, "Profile"=w186:u64, "ppx"=w185:sgl, "ppy"=w184:sgl, "fx"=w183:sgl, "fy"=w182:sgl, "model"=w181:u32, "index"=w180:u16)
    n36 = Equal?(x=w189, y=w188) -> (x = y?=w187:bool)
    n37 = Equal?(x=w192, y=w191) -> (x = y?=w190:bool)
    n38 = Equal?(x=w180, y=u16 0) -> (x = y?=w178:bool)
    n39 = Compound Arithmetic op=AND(w187, w190, w178) -> (w200:bool)
    n40 = case shown="True" w200 {
      tunnel: w199 -> [_ w215]
      tunnel: w198 -> [_ w214]
      tunnel: w197 -> [_ w213]
      tunnel: [w203 w217] -> w196
      tunnel: w195 -> [w203 w216]
      tunnel: [w202 w212] -> w194
      tunnel: w193 -> [w202 w204]
      tunnel: w186 -> [_ w211]
      tunnel: w185 -> [_ w210]
      tunnel: w184 -> [_ w209]
      tunnel: w183 -> [_ w208]
      tunnel: w182 -> [_ w207]
      tunnel: w181 -> [_ w206]
      frame False {
      }
      frame True {
        n41 = Bundle("width"=w215, "height"=w214, "fps"=w213, "Profile"=w211, "ppx"=w210, "ppy"=w209, "fx"=w208, "fy"=w207, "model"=w206) -> (w205:T3)  [unwired: 1 in]
        n42 = Build Array (concatenate)(w204, w205) -> (w212:T1)
        n43 = Format Into String(format string="%d x %d @%dfps", w215, w214, w213) -> (resulting string=w218:string)  [unwired: 2 in, 1 out]
        n44 = Build Array (concatenate)(w216, w218) -> (w217:string[])
      }
    }
  }
  n45 = for {
    tunnel: "Stream profile array" -> [w242] mode=indexing
    shift-right: [w237] -> w23
    shift-left: string[] [] -> [w236]
    shift-right: [w235] -> w25
    shift-left: w2 -> [w234]
    tunnel: w21 -> [w232]
    tunnel: w22 -> [_]
    # "Unrectified L"
    n46 = Unbundle By Name(w242) -> ("height"=w239:i32, "width"=w240:i32, "fps"=w238:i32, "RS Stream"=w233:u16, "Profile"=w230:u64, "ppx"=w224:sgl, "ppy"=w229:sgl, "fx"=w228:sgl, "fy"=w227:sgl, "model"=w223:u32, "index"=w221:u16)  [unwired: 1 out]
    n47 = Equal?(x=w233, y=w232) -> (x = y?=w231:bool)
    n48 = Equal?(x=w223, y=u16 0) -> (x = y?=w225:bool)
    n49 = Equal?(x=w221, y=u16 1) -> (x = y?=w220:bool)
    n50 = Compound Arithmetic op=AND(w231, w225, w220) -> (w241:bool)
    n51 = case shown="True" w241 {
      tunnel: w240 -> [_ w256]
      tunnel: w239 -> [_ w255]
      tunnel: w238 -> [_ w254]
      tunnel: [w244 w258] -> w237
      tunnel: w236 -> [w244 w257]
      tunnel: [w243 w253] -> w235
      tunnel: w234 -> [w243 w245]
      tunnel: w230 -> [_ w252]
      tunnel: w224 -> [_ w251]
      tunnel: w229 -> [_ w250]
      tunnel: w228 -> [_ w249]
      tunnel: w227 -> [_ w248]
      tunnel: w223 -> [_ w247]
      frame False {
      }
      frame True {
        n52 = Bundle("width"=w256, "height"=w255, "fps"=w254, "Profile"=w252, "ppx"=w251, "ppy"=w250, "fx"=w249, "fy"=w248, "model"=w247) -> (w246:T3)  [unwired: 1 in]
        n53 = Build Array (concatenate)(w245, w246) -> (w253:T1)
        n54 = Format Into String(format string="%d x %d @%dfps", w256, w255, w254) -> (resulting string=w259:string)  [unwired: 2 in, 1 out]
        n55 = Build Array (concatenate)(w257, w259) -> (w258:string[])
      }
    }
  }
  n56 = for {
    tunnel: "Stream profile array" -> [w283] mode=indexing
    shift-right: [w278] -> w16
    shift-left: string[] [] -> [w277]
    shift-right: [w276] -> w14
    shift-left: w2 -> [w275]
    tunnel: w18 -> [w273]
    tunnel: w17 -> [_]
    # "Unrectified L"
    n57 = Unbundle By Name(w283) -> ("height"=w280:i32, "width"=w281:i32, "fps"=w279:i32, "RS Stream"=w274:u16, "Profile"=w271:u64, "ppx"=w265:sgl, "ppy"=w270:sgl, "fx"=w269:sgl, "fy"=w268:sgl, "model"=w264:u32, "index"=w262:u16)  [unwired: 1 out]
    n58 = Equal?(x=w274, y=w273) -> (x = y?=w272:bool)
    n59 = Equal?(x=w264, y=u16 0) -> (x = y?=w266:bool)
    n60 = Equal?(x=w262, y=u16 2) -> (x = y?=w261:bool)
    n61 = Compound Arithmetic op=AND(w272, w266, w261) -> (w282:bool)
    n62 = case shown="True" w282 {
      tunnel: w281 -> [_ w297]
      tunnel: w280 -> [_ w296]
      tunnel: w279 -> [_ w295]
      tunnel: [w285 w299] -> w278
      tunnel: w277 -> [w285 w298]
      tunnel: [w284 w294] -> w276
      tunnel: w275 -> [w284 w286]
      tunnel: w271 -> [_ w293]
      tunnel: w265 -> [_ w292]
      tunnel: w270 -> [_ w291]
      tunnel: w269 -> [_ w290]
      tunnel: w268 -> [_ w289]
      tunnel: w264 -> [_ w288]
      frame False {
      }
      frame True {
        n63 = Bundle("width"=w297, "height"=w296, "fps"=w295, "Profile"=w293, "ppx"=w292, "ppy"=w291, "fx"=w290, "fy"=w289, "model"=w288) -> (w287:T3)  [unwired: 1 in]
        n64 = Build Array (concatenate)(w286, w287) -> (w294:T1)
        n65 = Format Into String(format string="%d x %d @%dfps", w297, w296, w295) -> (resulting string=w300:string)  [unwired: 2 in, 1 out]
        n66 = Build Array (concatenate)(w298, w300) -> (w299:string[])
      }
    }
  }
  n67 = for {
    tunnel: "Stream profile array" -> [w325] mode=indexing
    shift-right: [w320] -> w6
    shift-left: string[] [] -> [w319]
    shift-right: [w318] -> w8
    shift-left: w2 -> [w317]
    tunnel: w4 -> [w315]
    tunnel: w5 -> [w303]
    # "External RGB"
    n68 = Unbundle By Name(w325) -> ("height"=w322:i32, "width"=w323:i32, "fps"=w321:i32, "RS Stream"=w316:u16, "RS Format"=w304:u16, "Profile"=w313:u64, "ppx"=w309:sgl, "ppy"=w312:sgl, "fx"=w311:sgl, "fy"=w310:sgl, "model"=w308:u32, "index"=w306:u16)
    n69 = Equal?(x=w316, y=w315) -> (x = y?=w314:bool)
    n70 = Equal?(x=w306, y=u16 0) -> (x = y?=w305:bool)
    n71 = Equal?(x=w304, y=w303) -> (x = y?=w302:bool)
    n72 = Compound Arithmetic op=AND(w314, w305, w302) -> (w324:bool)
    n73 = case shown="True" w324 {
      tunnel: w323 -> [_ w339]
      tunnel: w322 -> [_ w338]
      tunnel: w321 -> [_ w337]
      tunnel: [w327 w341] -> w320
      tunnel: w319 -> [w327 w340]
      tunnel: [w326 w336] -> w318
      tunnel: w317 -> [w326 w328]
      tunnel: w313 -> [_ w335]
      tunnel: w309 -> [_ w334]
      tunnel: w312 -> [_ w333]
      tunnel: w311 -> [_ w332]
      tunnel: w310 -> [_ w331]
      tunnel: w308 -> [_ w330]
      frame False {
      }
      frame True {
        n74 = Bundle("width"=w339, "height"=w338, "fps"=w337, "Profile"=w335, "ppx"=w334, "ppy"=w333, "fx"=w332, "fy"=w331, "model"=w330) -> (w329:T3)  [unwired: 1 in]
        n75 = Build Array (concatenate)(w328, w329) -> (w336:T1)
        n76 = Format Into String(format string="%d x %d @%dfps", w339, w338, w337) -> (resulting string=w342:string)  [unwired: 2 in, 1 out]
        n77 = Build Array (concatenate)(w340, w342) -> (w341:string[])
      }
    }
  }
  n78 = Reverse 1D Array(array=w35) -> (reversed array=→"IR Left Array":string[])
  n79 = Reverse 1D Array(array=w37) -> (reversed array=→"IR left":T1)
  n80 = Reverse 1D Array(array=w46) -> (reversed array=→"Depth Stream":T1)
  n81 = Reverse 1D Array(array=w48) -> (reversed array=→"Depth Stream strings":string[])
  n82 = Reverse 1D Array(array=w25) -> (reversed array=→"Unrectified L IR":T1)
  n83 = Reverse 1D Array(array=w23) -> (reversed array=→"Unrectified L IR":string[])
  n84 = Reverse 1D Array(array=w14) -> (reversed array=→"Unrectified R  IR":T1)
  n85 = Reverse 1D Array(array=w16) -> (reversed array=→"Unrectified R IR":string[])
  n86 = Reverse 1D Array(array=w8) -> (reversed array=→"RGB ext.":T1)
  n87 = Reverse 1D Array(array=w6) -> (reversed array=→"RGB ext.":string[])
  n88 = Reverse 1D Array(array=w28) -> (reversed array=→"IR Right":T1)
  n89 = Reverse 1D Array(array=w30) -> (reversed array=→"IR Right Array":string[])
  n90 = Reverse 1D Array(array=w41) -> (reversed array=→"Color Left":T1)
  n91 = Reverse 1D Array(array=w43) -> (reversed array=→"Color Left Array":string[])
